vi "Demo Main_before_6_8_23_changes.vi"() -> ()   [LabVIEW 2022 SP3]
uses:
  Logo.ctl
  C:/Users/Public/OneDrive/Desktop/PMT program/SampleCodeLabView/Kinesis_with_LabVIEW_Examples_LV12 - v3/Thorlabs.MotionControl.Controls.dll
  Kinesis_with_LabVIEW_Examples_LV12 - v3/Thorlabs.MotionControl.Controls.dll
  <vilib>/Utility/file.llb/Write Delimited Spreadsheet (string).vi
  <vilib>/Utility/file.llb/Write Delimited Spreadsheet (I64).vi
  <vilib>/Utility/file.llb/Write Delimited Spreadsheet (DBL).vi
  C:/Users/Public/OneDrive/Desktop/PMT program/SampleCodeLabView/Kinesis_with_LabVIEW_Examples_LV12 - v3/ThorLabs.MotionControl.KCube.DCServoCLI.dll
  Kinesis_with_LabVIEW_Examples_LV12 - v3/ThorLabs.MotionControl.KCube.DCServoCLI.dll
  <vilib>/Analysis/NI_AALBase.lvlib
panel:
  in  "Save All Gate Data":bool
  out "ESD":i32=10000 caption="Steps\nAdded/Removed"
  in  "ES":i32 caption="Add /Remove \nSteps"
  out "Sweep Graph":u32[](graph)
  out "SM":i32 caption="Sweep\nMean"
  out "SN":i32 caption="Current Sweep Iteration"
  out "SND":i32 caption="Total No. of Sweeps"
  in  "Auto-Sweep":bool
  in  "P8":bool
  out "PC":i32 caption="Current \nPosition"
  out "WTD":i32=10000 caption="Wait Time (ms)\nRead Data"
  out "EPD":i32 caption="End Position\nRead Data"
  out "SPD":i32 caption="Start Position\nRead Data"
  out "SSD":i32 caption="Step Size\nRead Data"
  in  "SP":i32 caption="Start Position (degrees)\n Set Data"
  in  "WT":i32=10000 caption="Wait Time (ms)\n Set Data"
  in  "EP":i32 caption="End Position (degrees)\n Set Data"
  in  "P7":bool
  in  "SS":i32 caption="Step Size (degrees)\nSet Data"
  in  "Motor Controller\nSerialNumber":string="27261255"
  in  "KCubeDCServoControl":refnum<k24>(container)
  in  "Export":bool
  out "DB":u32[](array[numeric])
  out "OVL":bool caption="LED ON : Over Rang Data"
  out "OLD":i32
  out "GN":i32 caption="Gate Number"
  in  "Correction":bool=TRUE
  in  "Logo":T1
  out "Graph":u32[](graph)
  in  "Stop":bool
  in  "Start":bool
  in  "P6":bool
  out "RND":i32 caption="Read Number\nRead Data"
  in  "P5":bool
  in  "RN":i32=100 caption="Read Number\nSet Data"
  out "PowerD":i32 caption="Power\nRead Data"
  out "ITD":i32 caption="Internal Time\nRead Data"
  in  "P4":bool
  in  "P3":bool
  in  "IT":i32=100 caption="Internal Time\nSet Data"
  in  "P2":bool
  out "Handle Number":i32
  in  "P1":bool caption="Switch\nPower OFF/Power ON"
  in  "EXIT":bool
  # "pmt serial: 30430219"
  # "note: If you change angle between linear polarized light and half-wave plate by theta, the \npolarization after the wave plate is changed by twice theta. The code doesn't account for this.\nThis means we really need to go only to 180degrees, because at that point we have rotated the polarization by 360deg."
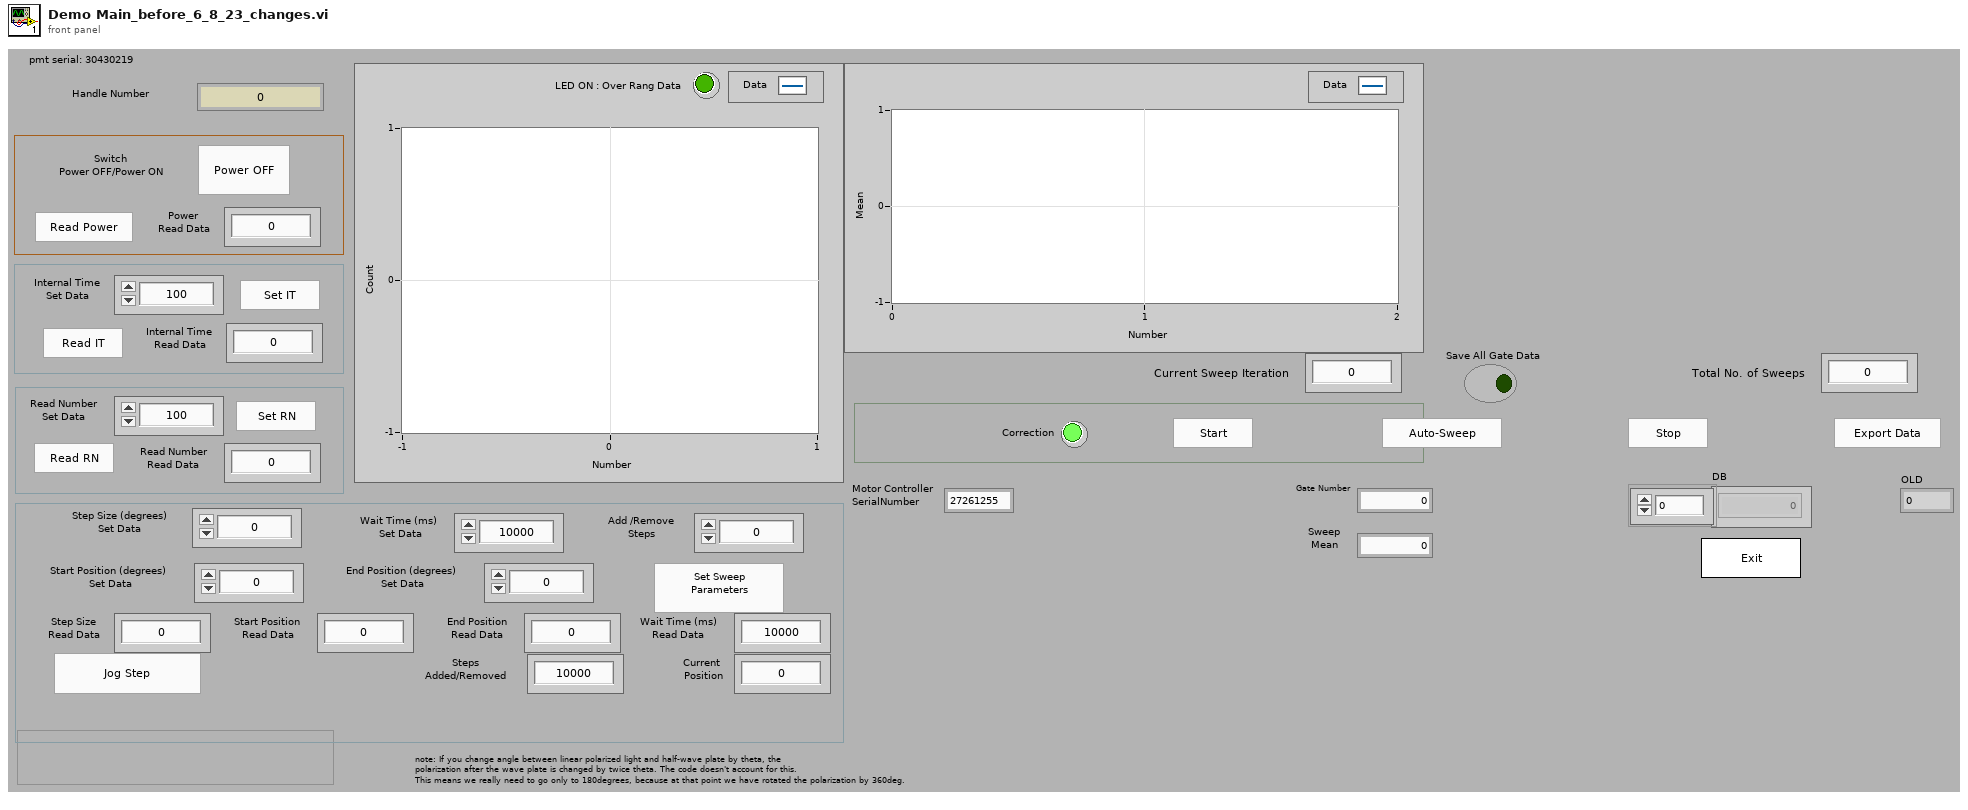
[diagram p1: front panel]
types:
  T1 = typedef "Logo.ctl" = bool
  T2 = enum8{"Enabled", "Disabled", "Disabled and Grayed Out"}
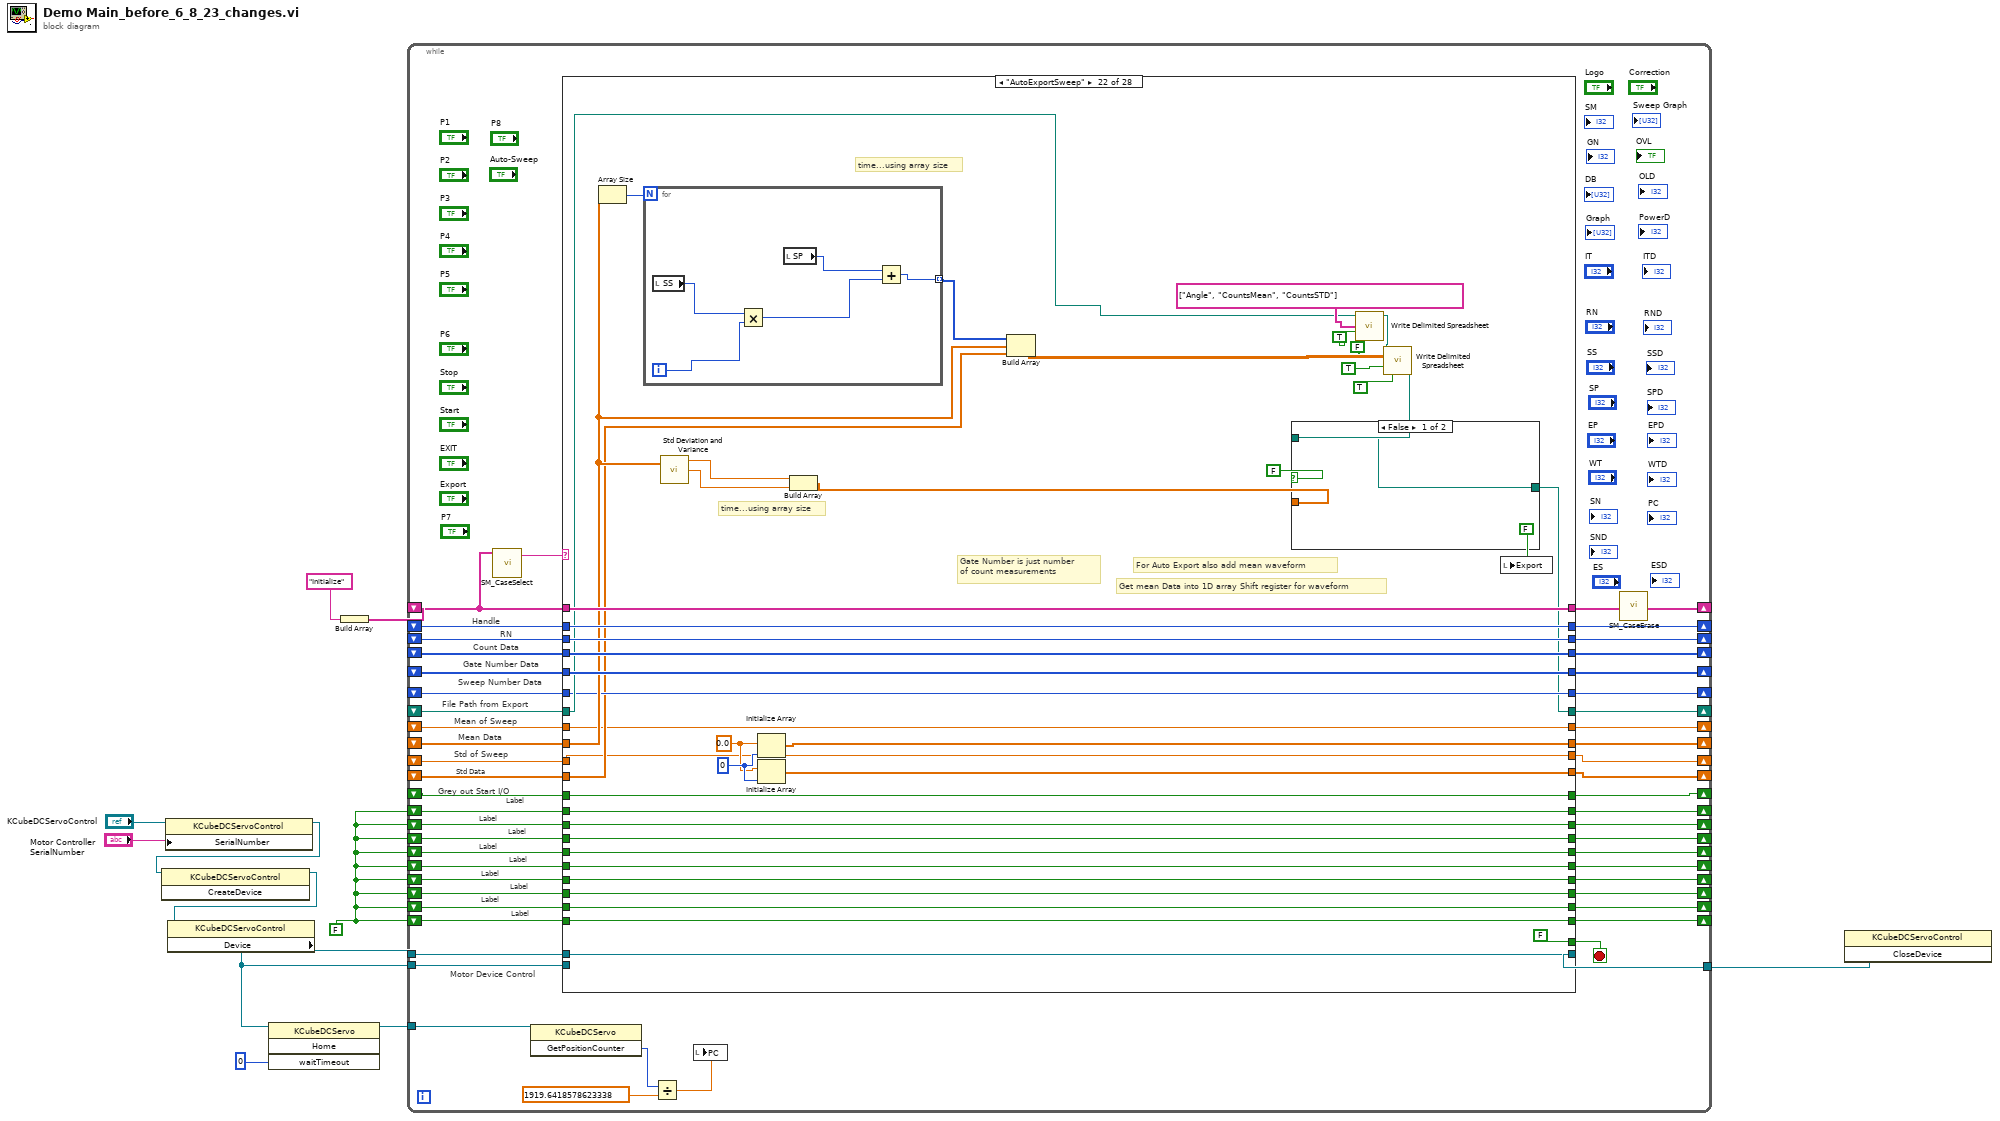
[diagram p0: block diagram]
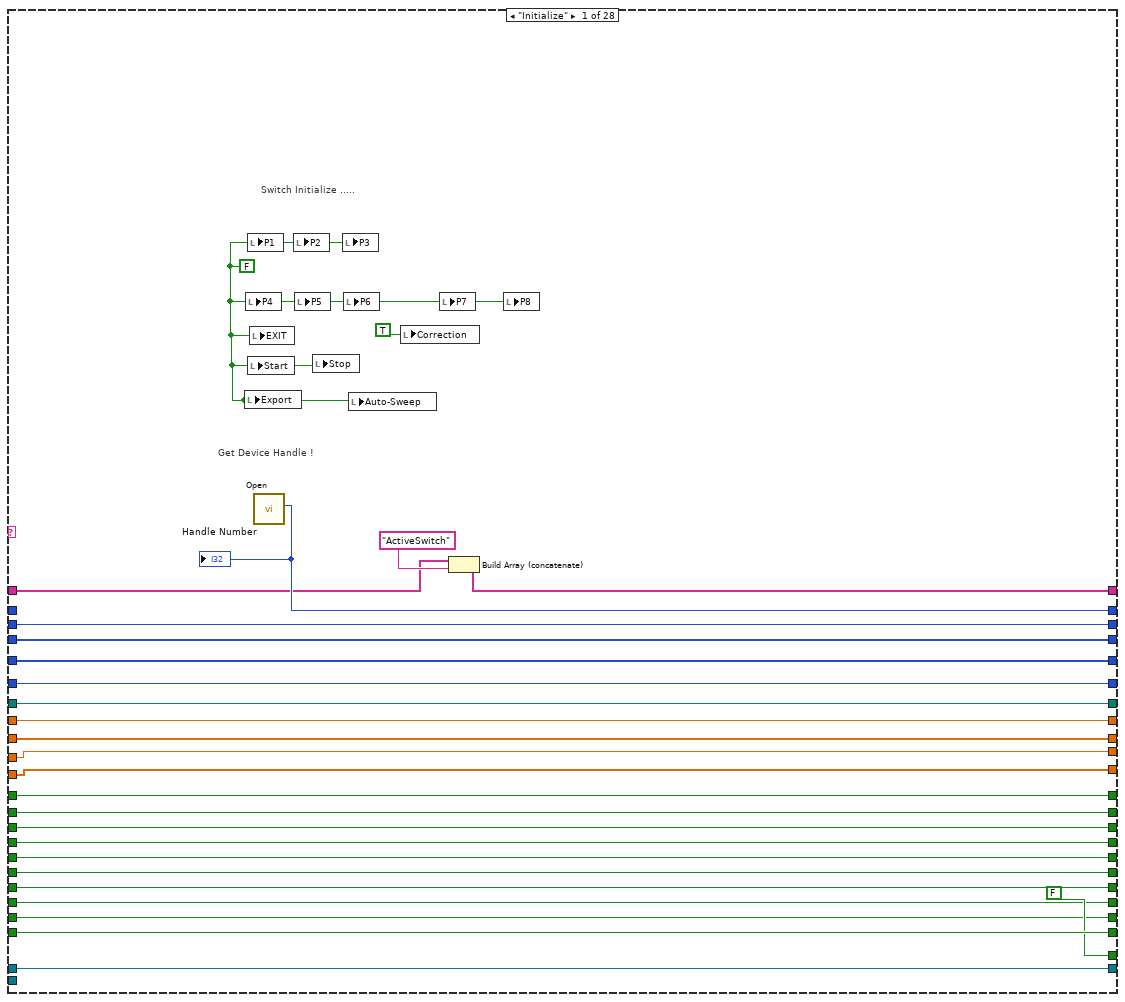
[diagram p2: hidden frame]
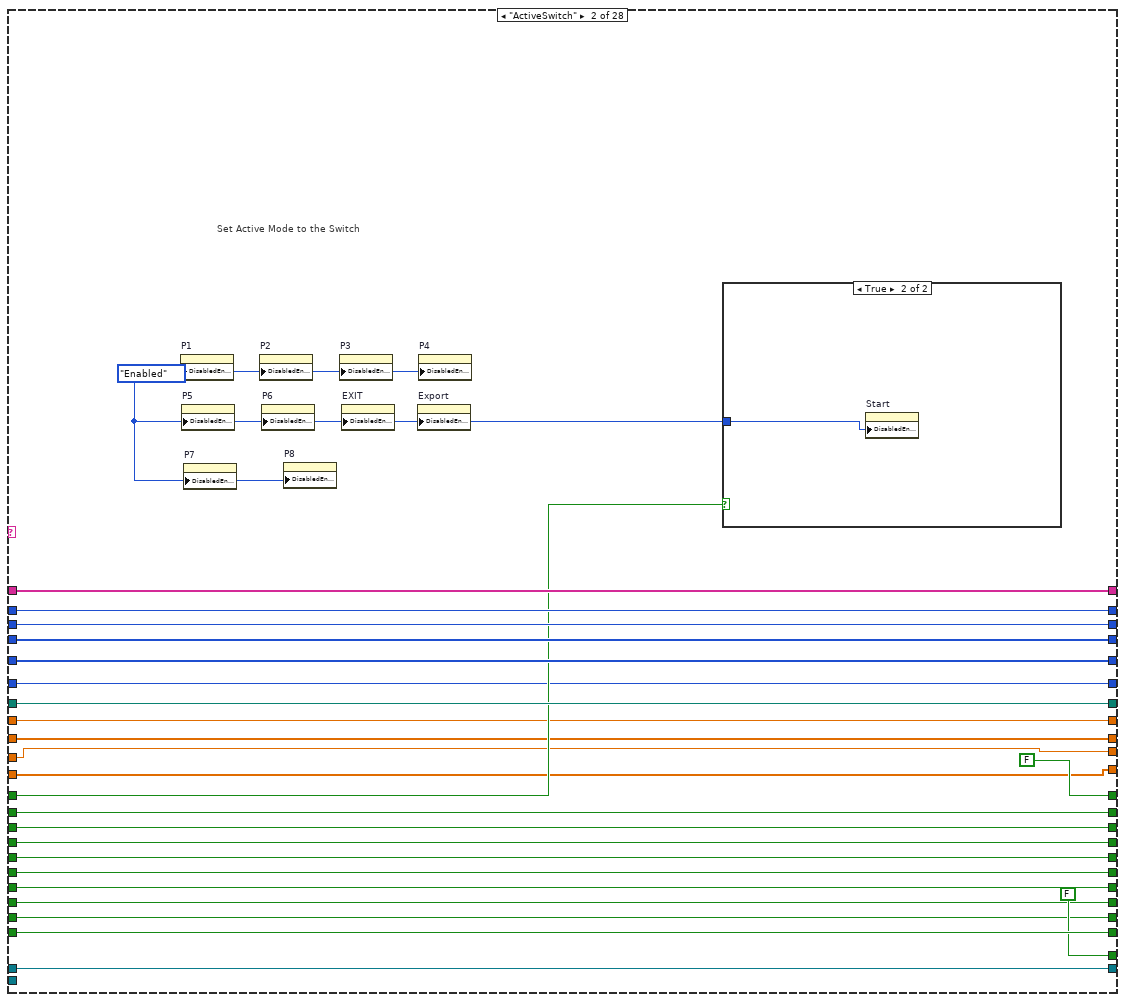
[diagram p3: hidden frame]
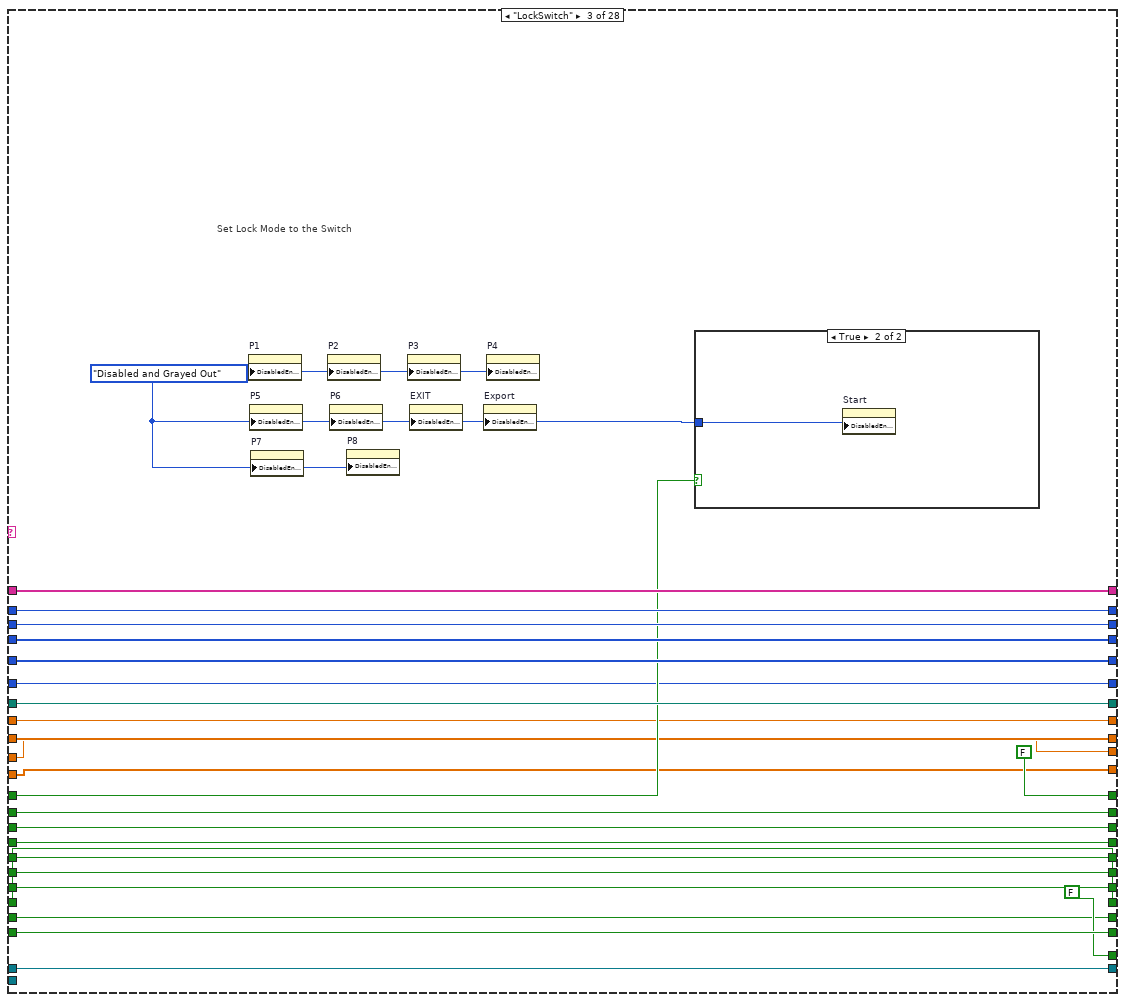
[diagram p5: hidden frame]
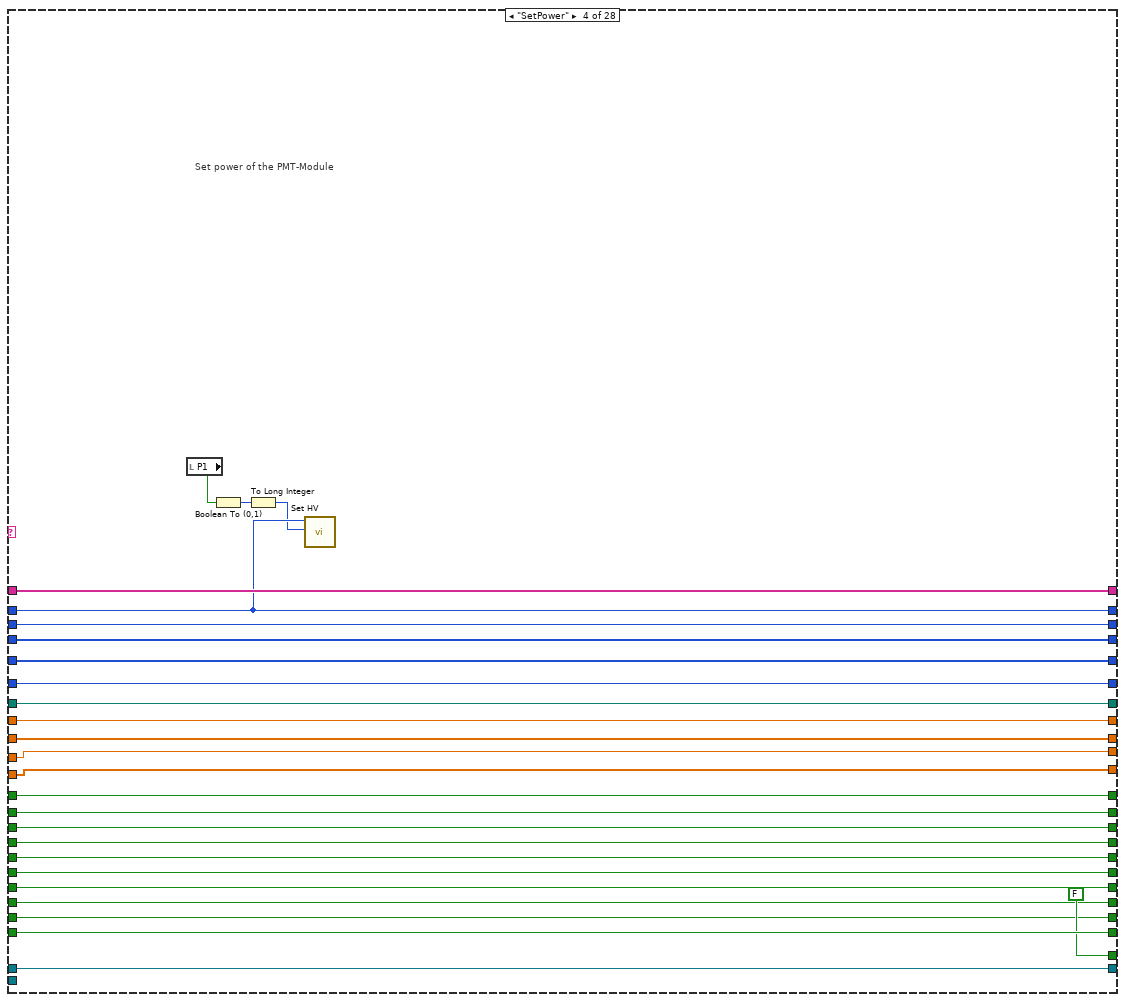
[diagram p7: hidden frame]
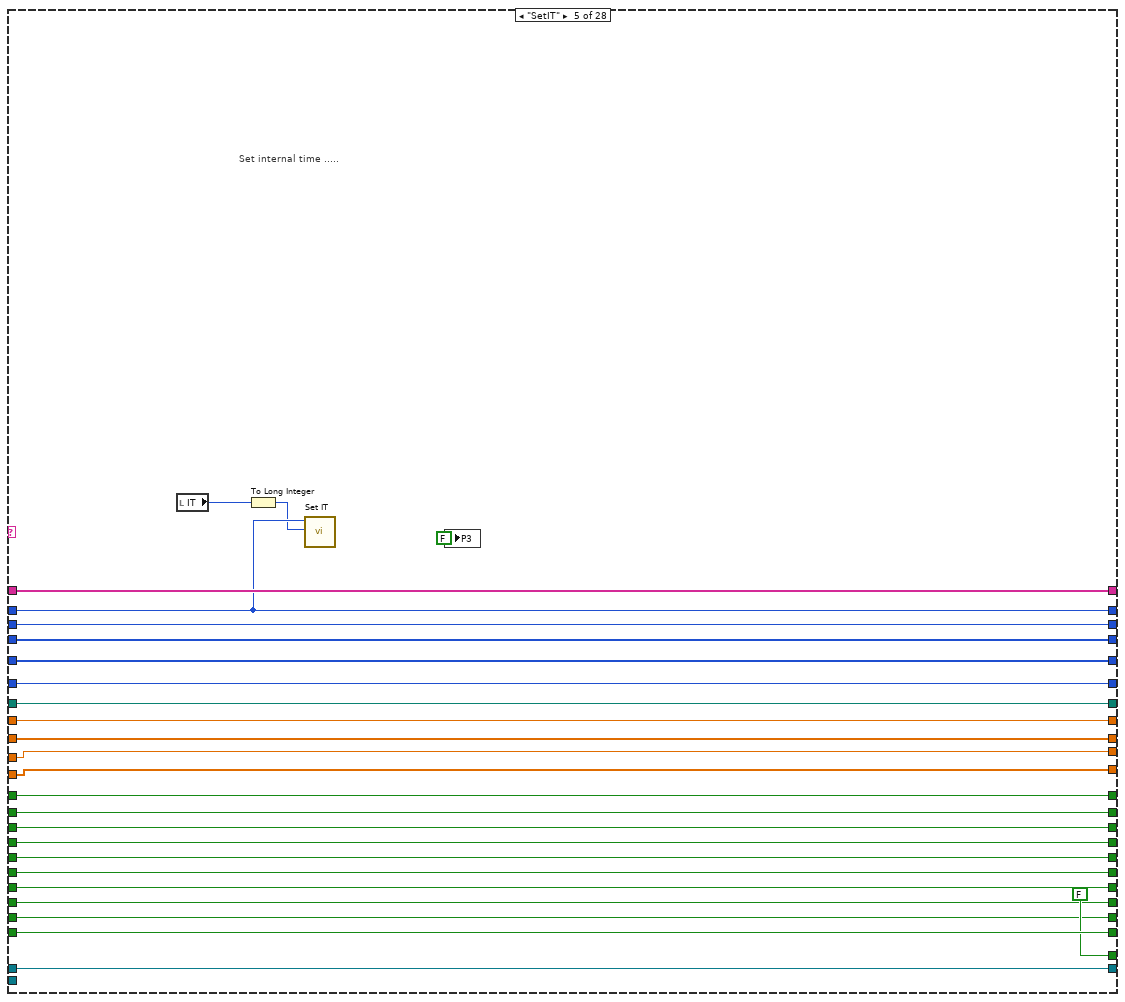
[diagram p8: hidden frame]
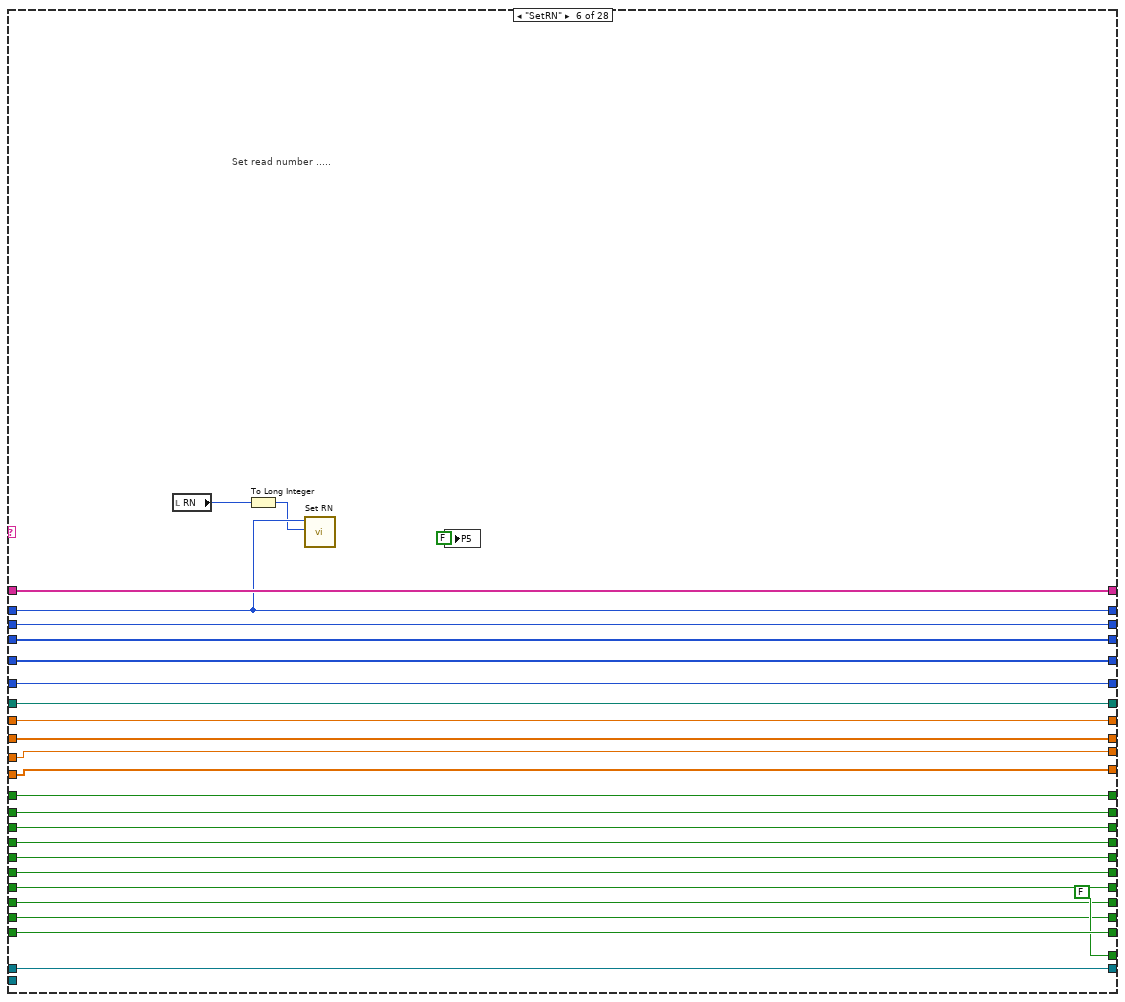
[diagram p9: hidden frame]
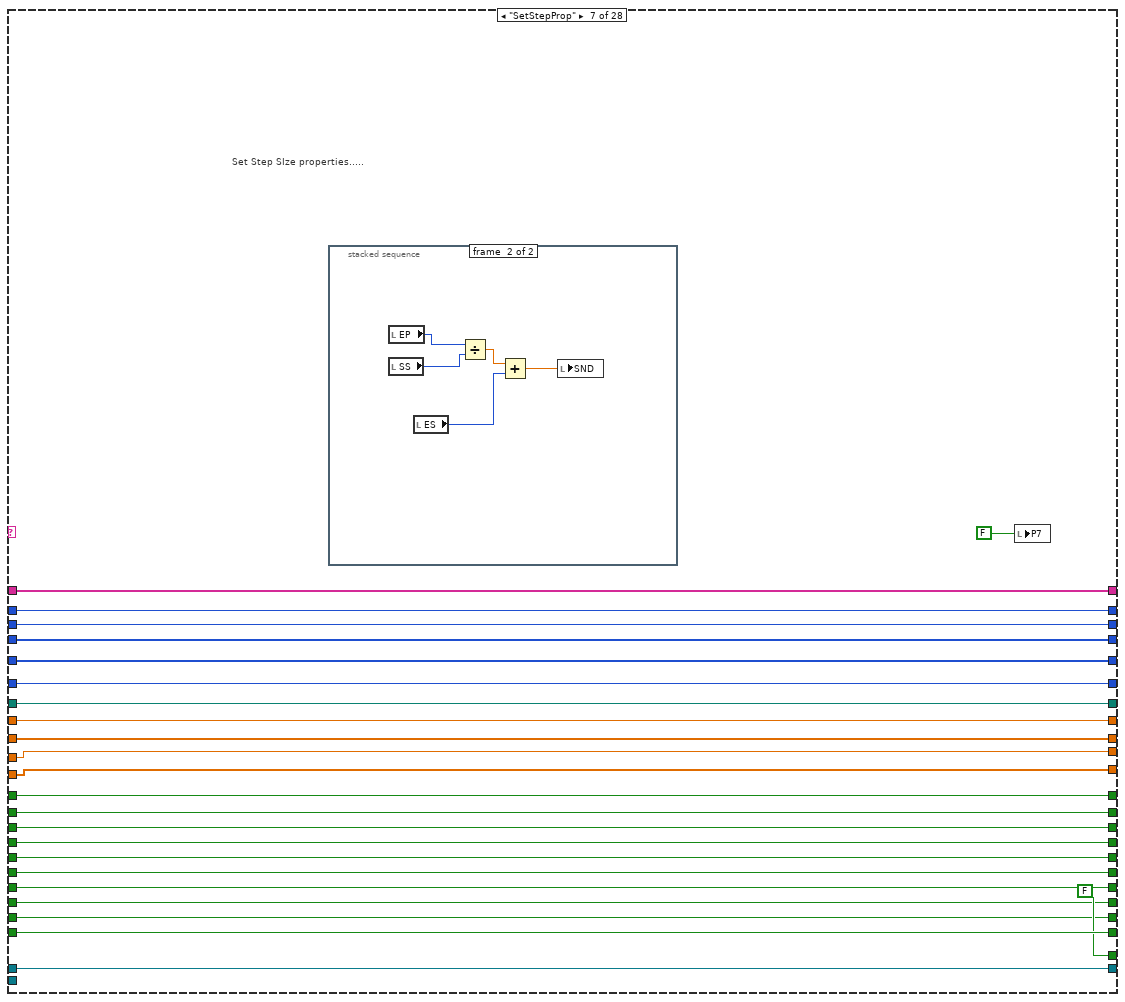
[diagram p10: hidden frame]
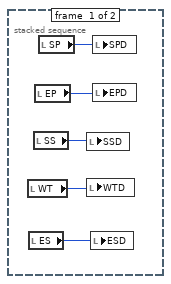
[diagram p11: hidden frame]
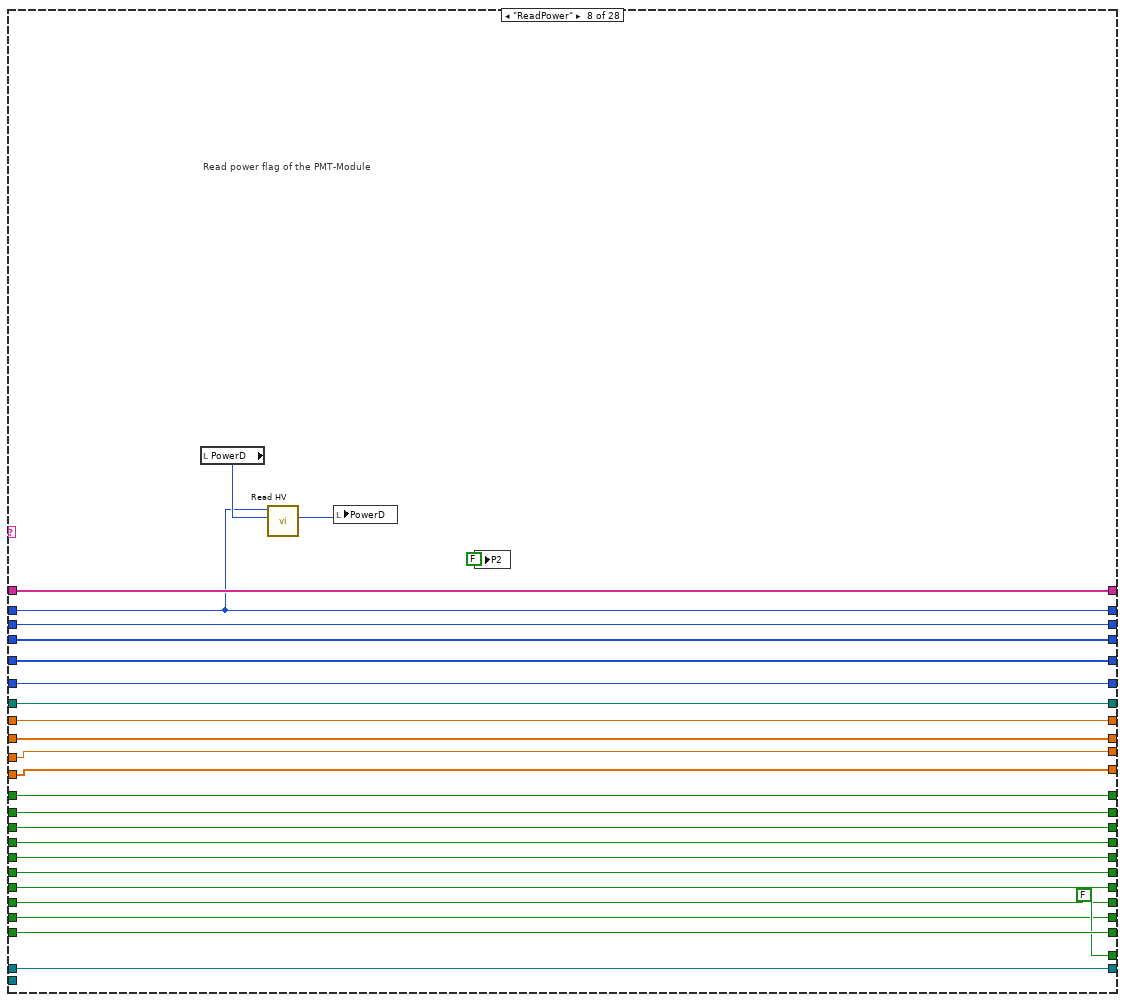
[diagram p12: hidden frame]
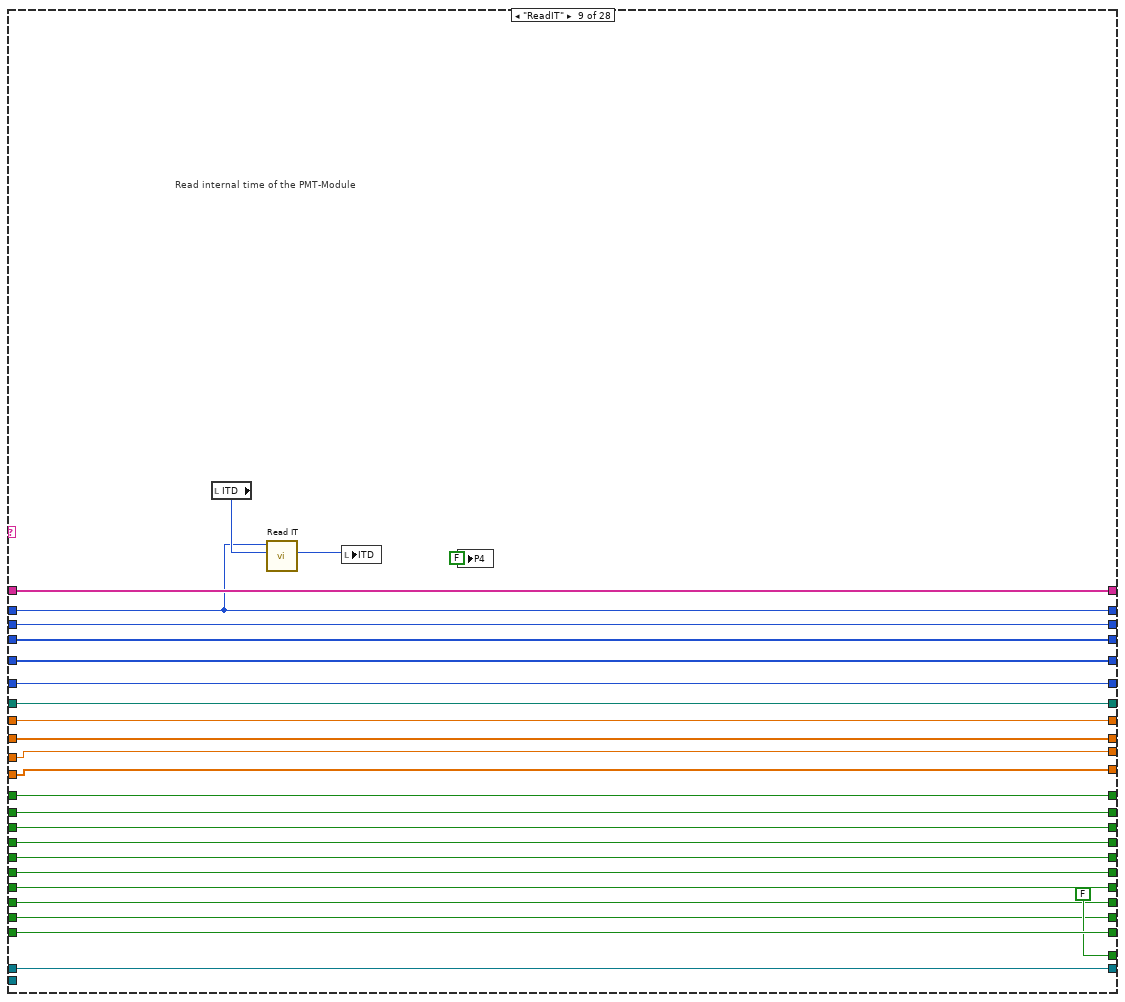
[diagram p13: hidden frame]
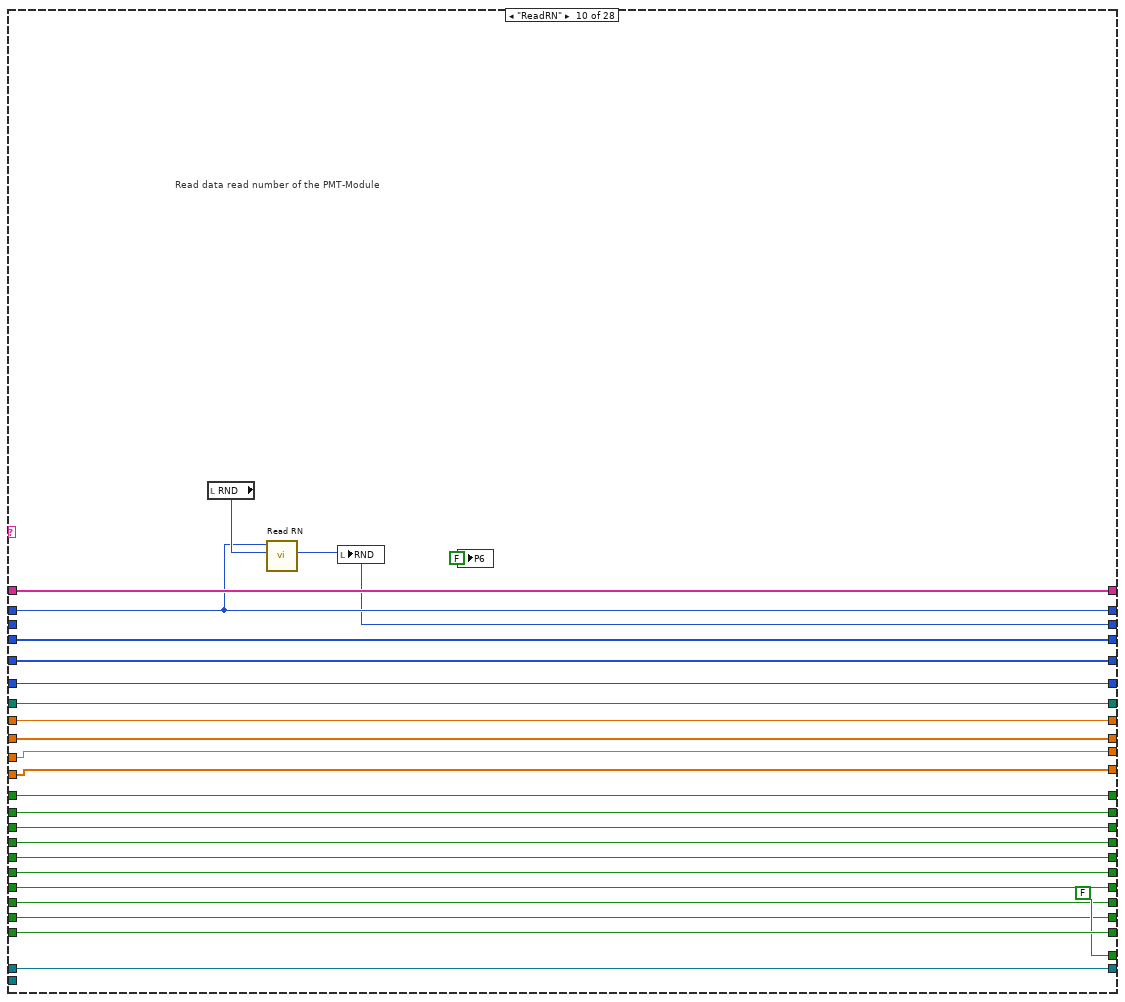
[diagram p14: hidden frame]
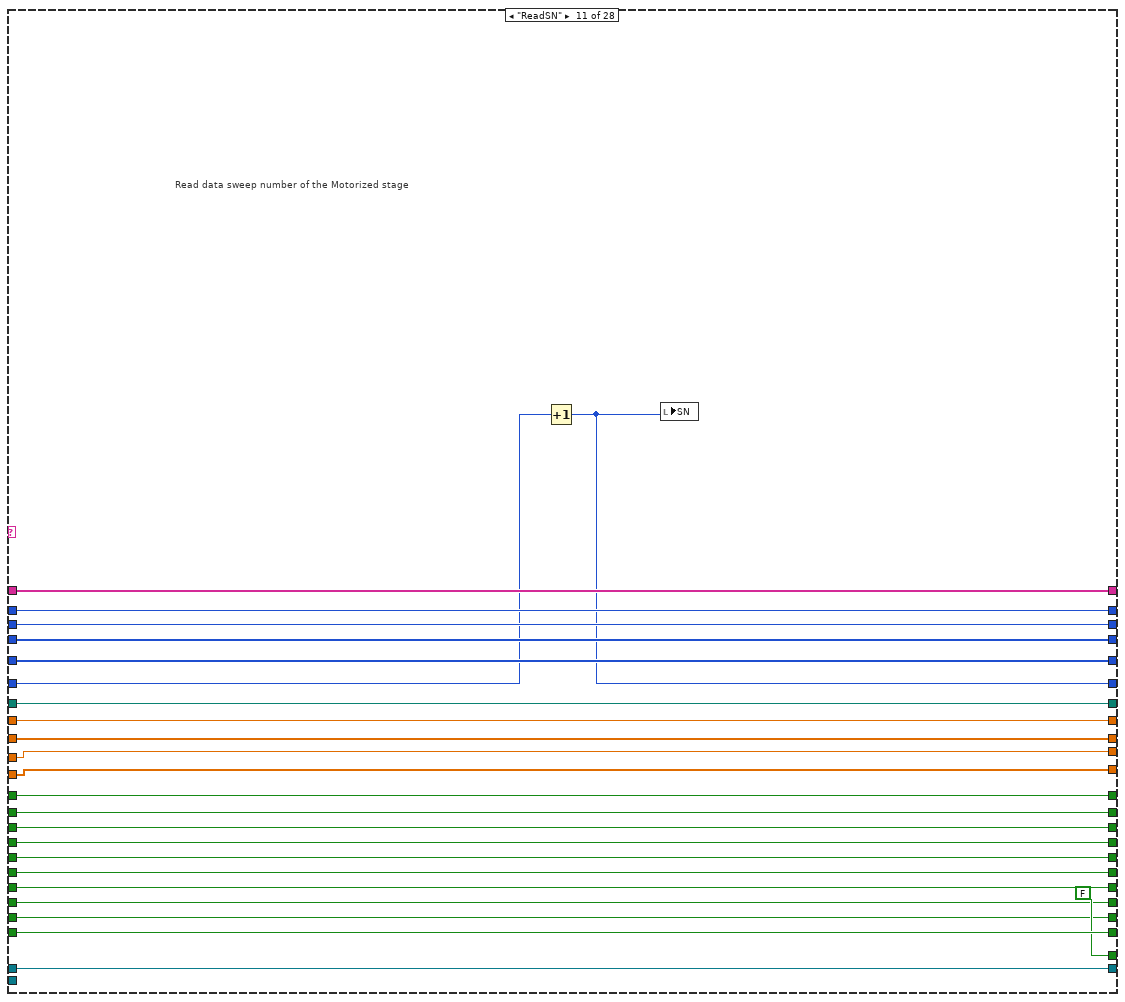
[diagram p15: hidden frame]
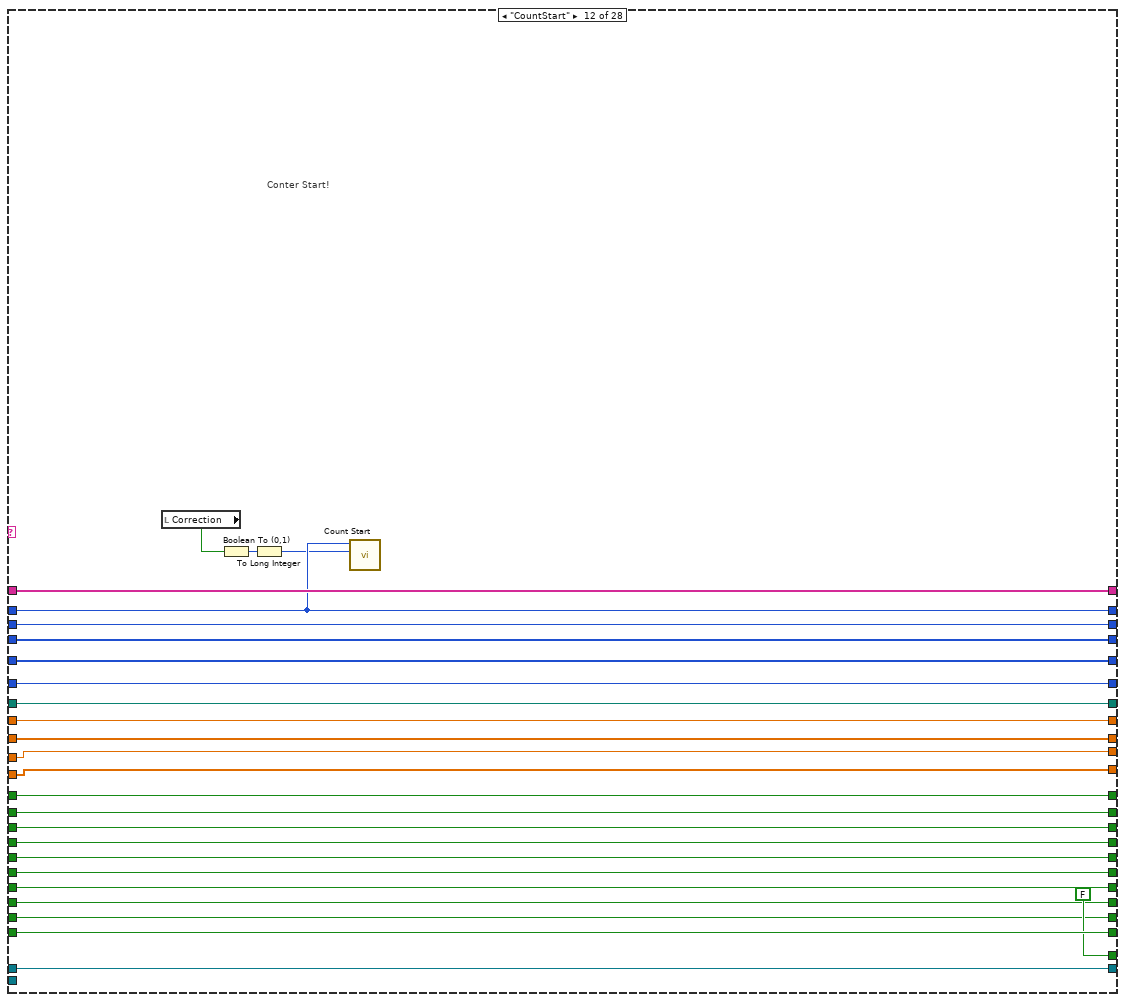
[diagram p16: hidden frame]
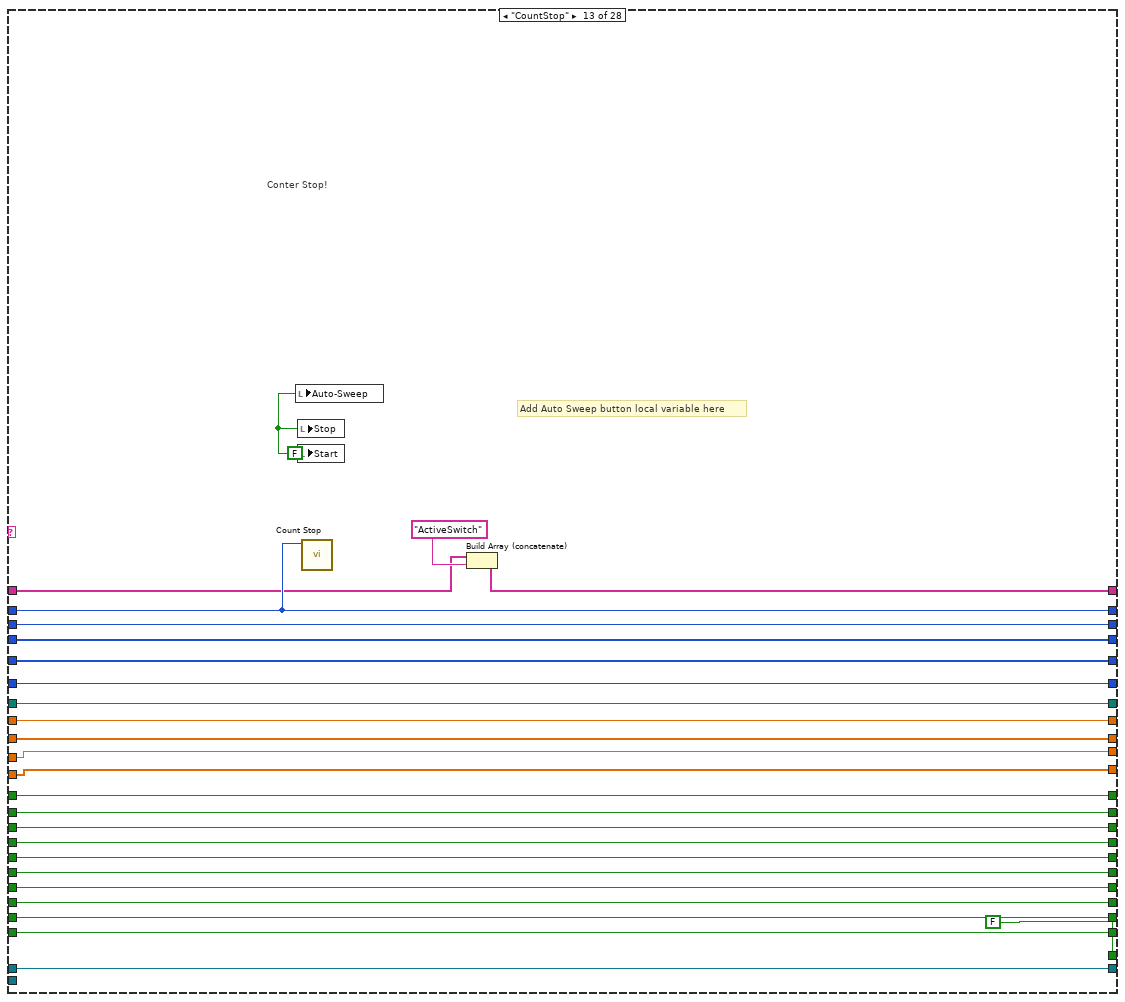
[diagram p17: hidden frame]
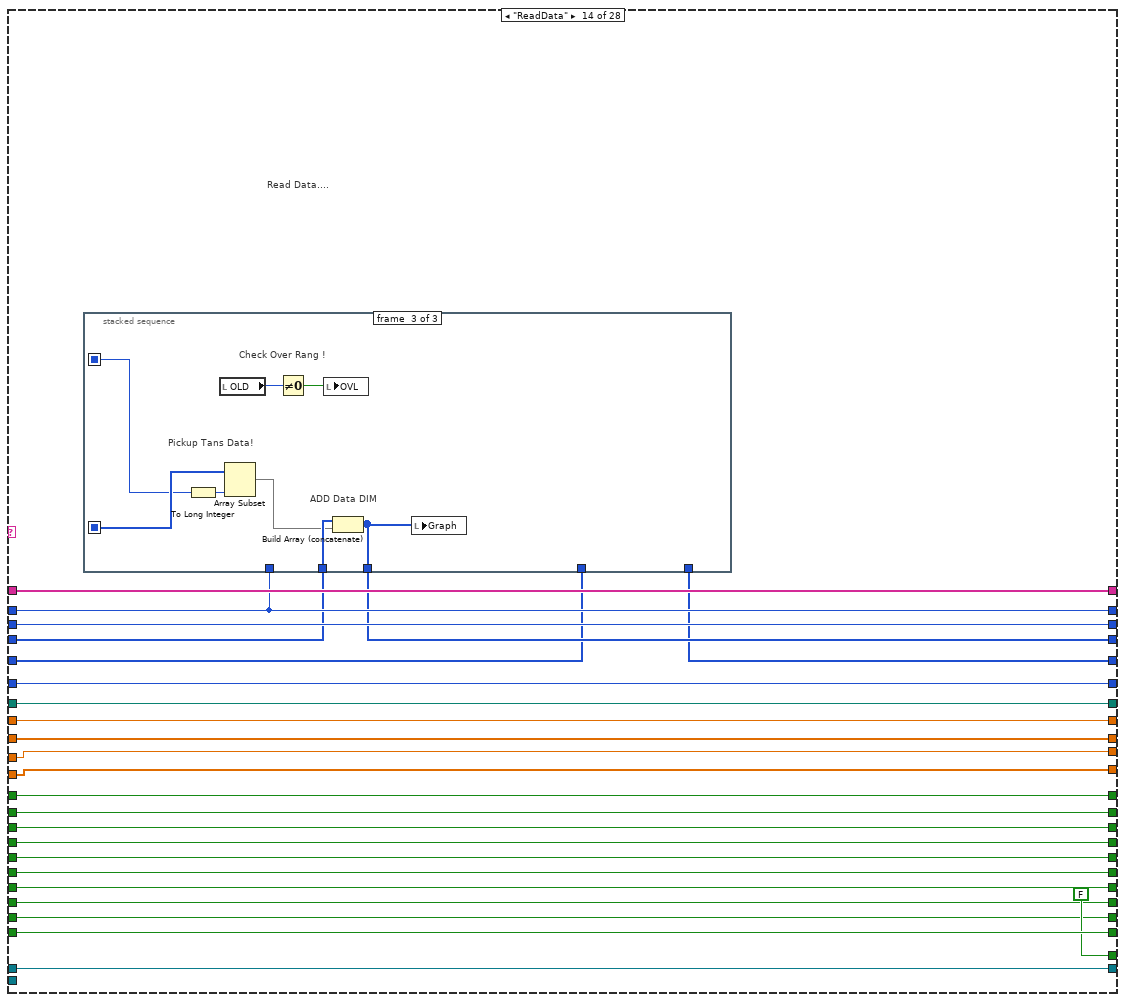
[diagram p18: hidden frame]
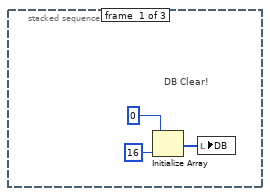
[diagram p19: hidden frame]
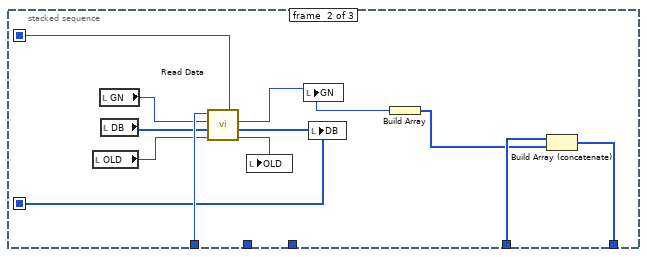
[diagram p20: hidden frame]
diagram:
  w10 = FALSE
  n1 = property class="KCubeDCServoControl"(reference="KCubeDCServoControl", "SerialNumber"="Motor Controller\nSerialNumber") -> (reference out=w8:refnum<k24>)  [unwired: 1 in, 1 out]
  n2 = invoke class="KCubeDCServoControl" method="CreateDevice"(reference=w8) -> (reference out=w1:refnum<k24>)  [unwired: 2 in, 2 out]
  n3 = property class="KCubeDCServoControl"(reference=w1) -> (reference out=w5:refnum<k24>, "Device"=w3:refnum<k24>)  [unwired: 1 in, 1 out]
  n4 = invoke class="KCubeDCServo" method="Home"(reference=w3, "waitTimeout"=0) -> (reference out=w2:refnum<k24>)  [unwired: 2 in, 3 out]
  n5 = Build Array("Initialize") -> (w11:string[])
  n6 = while {
    shift-right: [w47] -> _
    shift-left: w10 -> [w48]
    shift-right: [w49] -> _
    shift-left: w10 -> [w50]
    shift-right: [w51] -> _
    shift-left: w10 -> [w52]
    shift-right: [w53] -> _
    shift-left: w10 -> [w54]
    shift-right: [w55] -> _
    shift-left: _ -> [w56]
    shift-right: [w57] -> _
    shift-left: _ -> [w58]
    shift-right: [w59] -> _
    shift-left: _ -> [w60]
    shift-right: [w45] -> _
    shift-left: w10 -> [w46]
    shift-right: [w63] -> _
    shift-left: w10 -> [w64]
    shift-right: [w42] -> _
    shift-left: w11 -> [w61]
    shift-right: [w40] -> _
    shift-left: w10 -> [w41]
    shift-right: [w38] -> _
    shift-left: w10 -> [w39]
    shift-right: [w37] -> _
    shift-left: w10 -> [w36]
    tunnel: w5 -> [w33]
    tunnel: [w32] -> w6
    shift-right: [w35] -> _
    shift-left: _ -> [w34]
    tunnel: w3 -> [w31]
    shift-right: [w30] -> _
    shift-left: _ -> [w29]
    shift-right: [w28] -> _
    shift-left: _ -> [w27]
    tunnel: w2 -> [w26]
    shift-right: [w24] -> _
    shift-left: _ -> [w25]
    shift-right: [w23] -> _
    shift-left: _ -> [w22]
    shift-right: [w21] -> _
    shift-left: _ -> [w20]
    shift-right: [w15] -> _
    shift-left: _ -> [w16]
    shift-right: [w13] -> _
    shift-left: _ -> [w14]
    stop <- w44 stop-if-true
    # "Std Data"
    # "Std of Sweep"
    # "Mean Data"
    # "Mean of Sweep"
    # "Sweep Number Data"
    # "Grey out Start I/O"
    # "Motor Device Control"
    # "File Path from Export"
    # "Gate Number Data"
    # "Label"
    # "Label"
    # "Label"
    # "Label"
    # "Label"
    # "Label"
    # "Label"
    # "Label"
    # "Label"
    # "Count Data"
    # "RN"
    # "Handle"
    n7 = call "SM_CaseSelect.vi"("Input"=w61) -> ("Case"=w62:string)  [unwired: 10 out]
    n8 = invoke class="KCubeDCServo" method="GetPositionCounter"(reference=w26) -> ("GetPositionCounter"=w18:i32)  [unwired: 2 in, 2 out]
    n9 = case shown="\"AutoExportSweep\"" w62 {
      selector: w62 -> [_ _ _ _ _ _ _ _ _ _ _ _ _ _ _ _ _ _ _ _ _ _ _ _ _ _ w1015 _]
      tunnel: w64 -> [w91 w116 w142 w169 w195 w221 w245 w281 w307 w332 w356 w382 w408 w433 w480 w516 w544 w586 w626 w697 w736 w811 w853 w877 w911 w960 w1033 w1056]
      tunnel: [w91 w116 w142 w169 w195 w221 w245 w281 w307 w332 w356 w382 w408 w433 w480 w516 w544 w586 w626 w697 w736 w811 w853 w877 w911 w960 w1033 w1056] -> w63
      tunnel: w61 -> [w77 w115 w141 w168 w194 w220 w244 w280 w306 w331 w355 w381 w394 w432 w479 w504 w522 w573 w614 w708 w747 w822 w845 w890 w924 w948 w1032 w1055]
      tunnel: [w76 w115 w141 w168 w194 w220 w244 w280 w306 w331 w355 w381 w393 w432 w479 w503 w521 w574 w615 w708 w747 w822 w844 w890 w924 w945 w1032 w1055] -> w43
      tunnel: w60 -> [_ w103 w129 w156 w182 w208 w232 w267 w293 w319 w344 w369 w396 w421 w468 w505 w533 w576 w616 w707 w746 w821 w865 w889 w923 w959 w1031 w1043]
      tunnel: [w79 w103 w129 w156 w182 w208 w232 w267 w293 w319 w344 w369 w396 w421 w468 w505 w533 w576 w616 w707 w746 w821 w865 w889 w923 w959 w1031 w1043] -> w59
      tunnel: w58 -> [w90 w114 w140 w167 w193 w219 w243 w279 w305 _ w337 w380 w407 w431 w478 w515 w543 w571 w612 w706 w745 w820 w864 w888 w922 w958 w1030 w1054]
      tunnel: [w90 w114 w140 w167 w193 w219 w243 w279 w305 w317 w337 w380 w407 w431 w478 w515 w543 w571 w612 w706 w745 w820 w864 w888 w922 w958 w1030 w1054] -> w57
      tunnel: w56 -> [w89 w113 w139 w166 w192 w218 w242 w278 w304 w330 w354 w379 w406 w420 w463 _ _ w567 w610 w682 w731 w801 w863 w887 w921 w944 w1029 w1053]
      tunnel: [w89 w113 w139 w166 w192 w218 w242 w278 w304 w330 w354 w379 w406 w419 w463 w495 w531 w567 w610 w682 w731 w801 w863 w887 w921 w944 w1029 w1053] -> w55
      tunnel: w54 -> [w88 w112 w138 w165 w191 w217 w241 w277 w303 w329 w353 w378 w405 w430 w477 w514 w542 w585 w625 w705 w744 w819 w861 w885 w919 w957 w1028 w1052]
      tunnel: [w88 w112 w138 w165 w191 w217 w241 w277 w303 w329 w353 w378 w405 w430 w477 w514 w542 w585 w625 w705 w744 w819 w861 w885 w919 w957 w1028 w1052] -> w53
      tunnel: w52 -> [w87 w111 w137 w164 w190 w216 w240 w276 w302 w328 w352 w377 w404 w429 w476 w513 w541 w584 w624 w704 w743 w818 w860 w884 w918 w956 w1027 w1051]
      tunnel: [w87 w111 w137 w164 w190 w216 w240 w276 w302 w328 w352 w377 w404 w429 w476 w513 w541 w584 w624 w704 w743 w818 w860 w884 w918 w956 w1027 w1051] -> w51
      tunnel: w50 -> [w86 w110 w136 w163 w189 w215 w239 w275 w301 w327 w351 w376 w403 w428 w475 w512 w540 w583 w623 w703 w742 w817 w859 w883 w917 w955 w1026 w1050]
      tunnel: [w86 w110 w136 w163 w189 w215 w239 w275 w301 w327 w351 w376 w403 w428 w475 w512 w540 w583 w623 w703 w742 w817 w859 w883 w917 w955 w1026 w1050] -> w49
      tunnel: w48 -> [w85 w109 w135 w162 w188 w214 w238 w274 w300 w326 w350 w375 w402 w427 w474 w511 w539 w582 w622 w702 w741 w816 w858 w882 w916 w954 w1025 w1049]
      tunnel: [w85 w109 w135 w162 w188 w214 w238 w274 w300 w326 w350 w375 w402 w427 w474 w511 w539 w582 w622 w702 w741 w816 w858 w882 w916 w954 w1025 w1049] -> w47
      tunnel: w46 -> [w84 w108 w134 w161 w187 w213 w237 w273 w299 w325 w349 w374 w401 w426 w473 w510 w538 w581 w621 w701 w740 w815 w857 w881 w915 w953 w1024 w1048]
      tunnel: [w84 w108 w134 w161 w187 w213 w237 w273 w299 w325 w349 w374 w401 w426 w473 w510 w538 w581 w621 w701 w740 w815 w857 w881 w915 w953 w1024 w1048] -> w45
      tunnel: [FALSE FALSE FALSE FALSE FALSE FALSE FALSE FALSE FALSE FALSE FALSE FALSE FALSE FALSE FALSE FALSE FALSE FALSE FALSE FALSE FALSE FALSE FALSE FALSE FALSE FALSE FALSE TRUE] -> w44
      tunnel: w41 -> [w80 w104 w130 w157 w183 w209 w233 w269 w295 w321 w345 w370 w397 w422 w469 w506 w534 w577 w617 w700 w739 w814 w856 w880 w914 w949 w1020 w1044]
      tunnel: [w80 w104 w130 w157 w183 w209 w233 w269 w295 w321 w345 w370 w397 w422 w469 w506 w534 w577 w617 w700 w739 w814 w856 w880 w914 w949 w1020 w1044] -> w40
      tunnel: w39 -> [w82 w106 w132 w159 w185 w211 w235 w271 w297 w323 w347 w372 w399 w424 w471 w508 w536 w579 w619 w699 w738 w813 w855 w879 w913 w951 w1022 w1046]
      tunnel: [w82 w106 w132 w159 w185 w211 w235 w271 w297 w323 w347 w372 w399 w424 w471 w508 w536 w579 w619 w699 w738 w813 w855 w879 w913 w951 w1022 w1046] -> w38
      tunnel: [w81 w105 w131 w158 w184 w210 w234 w270 w296 w322 w346 w371 w398 w423 w470 w507 w535 w578 w618 w698 w737 w812 w854 w878 w912 w950 w1021 w1045] -> w37
      tunnel: w36 -> [w81 w105 w131 w158 w184 w210 w234 w270 w296 w322 w346 w371 w398 w423 w470 w507 w535 w578 w618 w698 w737 w812 w854 w878 w912 w950 w1021 w1045]
      tunnel: [w75 w102 w128 w152 w178 w204 w231 w264 w290 w316 w343 w365 w392 w418 w462 w495 w531 w566 w609 w677 w717 w796 w862 w886 w920 w943 w1014 w1042] -> w35
      tunnel: w34 -> [w75 w102 w128 w152 w178 w204 w231 w264 w290 w316 w343 w365 w392 w417 w462 _ _ w566 w609 w677 w717 w796 w862 w886 w920 w943 w1014 w1042]
      tunnel: w33 -> [w74 w101 w127 w151 w177 w203 w230 w263 w289 w315 w342 w364 w391 w416 w467 w494 w530 w565 w608 w679 w729 w798 w852 w876 w910 w942 w1013 w1041]
      tunnel: [w74 w101 w127 w151 w177 w203 w230 w263 w289 w315 w342 w364 w391 w416 w467 w494 w530 w565 w608 w679 w729 w798 w852 w876 w910 w942 w1013 w1041] -> w32
      tunnel: w31 -> [_ _ _ _ _ _ _ _ _ _ _ _ _ _ _ _ _ _ _ _ _ _ _ w873 w907 _ _ _]
      tunnel: [w73 w100 w126 w150 w176 w202 w228 w262 w288 w314 w341 w363 w390 w415 w466 w493 w529 w564 w607 w670 w727 w780 w841 w874 w908 w941 w1012 w1040] -> w30
      tunnel: w29 -> [w73 w100 w126 w150 w176 w202 w228 w262 w288 w314 w341 w363 w390 w415 w466 w493 w529 w564 w607 w670 w723 w794 _ w874 w908 w941 w1012 w1040]
      tunnel: [w72 FALSE FALSE w149 w175 w201 w227 w261 w287 w313 w340 w362 w389 w414 w465 w492 TRUE w563 w606 w672 w726 w795 w850 w872 w906 w940 w1011 w1039] -> w28
      tunnel: w27 -> [w72 w99 w125 w149 w175 w201 w227 w261 w287 w313 w340 w362 w389 w414 w465 w492 _ w563 _ w672 w726 w795 w850 w872 w906 w940 w1011 w1039]
      tunnel: w25 -> [w70 w96 w122 w148 w174 w200 w226 w260 w286 w312 w335 w361 w388 w413 w464 w491 w527 w562 w605 w671 w722 w791 _ w868 w905 w939 w1010 w1038]
      tunnel: [w70 w96 w122 w148 w174 w200 w226 w260 w286 w312 w336 w361 w388 w413 w464 w491 w527 w562 w605 w671 w722 w791 w842 w868 w905 w939 w1010 w1038] -> w24
      tunnel: [w69 w95 w121 w147 w173 w199 w225 w259 w285 w311 w339 w360 w387 w412 w461 w490 w526 w561 w602 w669 w725 w784 w849 w870 w904 w938 w1009 w1037] -> w23
      tunnel: w22 -> [w69 w95 w121 w147 w173 w199 w225 w259 w285 w311 w339 w360 w387 w412 w461 w490 w526 w561 w602 w669 _ w784 w849 w870 w904 w938 w1009 w1037]
      tunnel: [w68 w94 w120 w146 w172 w198 w224 w258 w284 w310 w338 w359 w386 w411 w460 w489 w525 w560 w601 w668 w724 w790 w843 w869 w903 w937 w1008 w1036] -> w21
      tunnel: w20 -> [w68 w94 w120 w146 w172 w198 w224 w258 w284 w310 w338 w359 w386 w411 w459 w489 w525 w560 w601 w668 w724 w792 w843 w869 w903 w937 w1008 w1036]
      tunnel: w16 -> [w67 w93 w119 w145 w171 w197 w223 w257 w283 w309 w334 w358 w384 w410 w458 w488 w518 w559 w599 w667 w716 w786 w839 w867 w902 w936 w1007 w1035]
      tunnel: [w67 w93 w119 w145 w171 w197 w223 w257 w283 w309 w334 w358 w384 w410 w456 w488 w518 w559 w599 w667 w716 w787 w839 w867 w902 w936 w1007 w1035] -> w15
      tunnel: w14 -> [w66 w92 w118 w144 w170 w196 w222 w256 w282 w308 w333 w357 w383 w409 w457 w487 w517 w558 w598 w666 _ w783 w838 w866 w901 w935 w1006 w1034]
      tunnel: [w66 w92 w118 w144 w170 w196 w222 w256 w282 w308 w333 w357 w383 w409 w457 w487 w517 w558 w598 w666 w715 w783 w838 w866 w901 w935 w1006 w1034] -> w13
      frame "Initialize" {
        w71 = FALSE ("P1")
        # "Get Device Handle !"
        # "Switch Initialize ....."
        n10 = local write "Export"(w71) -> ()
        n11 = local write "P4"(w71) -> ()
        n12 = local write "P1"(w71) -> ()
        n13 = local write "Start"(w71) -> ()
        n14 = local write "EXIT"(w71) -> ()
        n15 = call "Open.vi"() -> ("Handle Number"=w79:i32)  [unwired: 10 in, 1 out]
        "Handle Number" <- w79
        n16 = local write "P2"(w71) -> ()
        n17 = local write "P5"(w71) -> ()
        n18 = local write "Stop"(w71) -> ()
        n19 = local write "P3"(w71) -> ()
        n20 = local write "P6"(w71) -> ()
        n21 = local write "Auto-Sweep"(w71) -> ()
        n22 = local write "Correction"(TRUE ("P1")) -> ()
        n23 = local write "P7"(w71) -> ()
        n24 = Build Array (concatenate)(w77, "ActiveSwitch") -> (w76:string[])
        n25 = local write "P8"(w71) -> ()
      }
      frame "ActiveSwitch" {
        w97 = T2."Enabled" ("無効")
        # "Set Active Mode to the Switch"
        n26 = property on="P1" class="Bool (strict)"("DisabledEnum"=w97) -> ()  [unwired: 2 in, 2 out]
        n27 = property on="P5" class="Bool (strict)"("DisabledEnum"=w97) -> ()  [unwired: 2 in, 2 out]
        n28 = property on="P7" class="Bool (strict)"("DisabledEnum"=w97) -> ()  [unwired: 2 in, 2 out]
        n29 = property on="P2" class="Bool (strict)"("DisabledEnum"=w97) -> ()  [unwired: 2 in, 2 out]
        n30 = property on="P6" class="Bool (strict)"("DisabledEnum"=w97) -> ()  [unwired: 2 in, 2 out]
        n31 = property on="P8" class="Bool (strict)"("DisabledEnum"=w97) -> ()  [unwired: 2 in, 2 out]
        n32 = property on="P3" class="Bool (strict)"("DisabledEnum"=w97) -> ()  [unwired: 2 in, 2 out]
        n33 = property on="EXIT" class="Bool (strict)"("DisabledEnum"=w97) -> ()  [unwired: 2 in, 2 out]
        n34 = property on="Export" class="Bool (strict)"("DisabledEnum"=w97) -> ()  [unwired: 2 in, 2 out]
        n35 = property on="P4" class="Bool (strict)"("DisabledEnum"=w97) -> ()  [unwired: 2 in, 2 out]
        n36 = case shown="True" w99 {
          tunnel: w97 -> [_ w117]
          frame False {
          }
          frame True {
            n37 = property on="Start" class="Bool (strict)"("DisabledEnum"=w117) -> ()  [unwired: 2 in, 2 out]
          }
        }
      }
      frame "LockSwitch" {
        w123 = T2."Disabled and Grayed Out" ("無効")
        # "Set Lock Mode to the Switch"
        n38 = property on="P1" class="Bool (strict)"("DisabledEnum"=w123) -> ()  [unwired: 2 in, 2 out]
        n39 = property on="P5" class="Bool (strict)"("DisabledEnum"=w123) -> ()  [unwired: 2 in, 2 out]
        n40 = property on="P7" class="Bool (strict)"("DisabledEnum"=w123) -> ()  [unwired: 2 in, 2 out]
        n41 = property on="P2" class="Bool (strict)"("DisabledEnum"=w123) -> ()  [unwired: 2 in, 2 out]
        n42 = property on="P6" class="Bool (strict)"("DisabledEnum"=w123) -> ()  [unwired: 2 in, 2 out]
        n43 = property on="P8" class="Bool (strict)"("DisabledEnum"=w123) -> ()  [unwired: 2 in, 2 out]
        n44 = property on="P3" class="Bool (strict)"("DisabledEnum"=w123) -> ()  [unwired: 2 in, 2 out]
        n45 = property on="EXIT" class="Bool (strict)"("DisabledEnum"=w123) -> ()  [unwired: 2 in, 2 out]
        n46 = property on="Export" class="Bool (strict)"("DisabledEnum"=w123) -> ()  [unwired: 2 in, 2 out]
        n47 = property on="P4" class="Bool (strict)"("DisabledEnum"=w123) -> ()  [unwired: 2 in, 2 out]
        n48 = case shown="True" w125 {
          tunnel: w123 -> [_ w143]
          frame False {
          }
          frame True {
            n49 = property on="Start" class="Bool (strict)"("DisabledEnum"=w143) -> ()  [unwired: 2 in, 2 out]
          }
        }
      }
      frame "SetPower" {
        # "Set power of the PMT-Module"
        n50 = local read "P1"() -> (w155:bool)
        n51 = Boolean To (0,1)(Boolean=w155) -> (0, 1=w154:i16)
        n52 = To Long Integer(number=w154) -> (32bit integer=w153:i32)
        n53 = call "Set HV.vi"("HV"=w153, "handle"=w156) -> ()  [unwired: 8 in, 2 out]
      }
      frame "SetIT" {
        # "Set internal time ....."
        n54 = local read "IT"() -> (w180:i32)
        n55 = To Long Integer(number=w180) -> (32bit integer=w181:i32)
        n56 = call "Set IT.vi"("IT"=w181, "handle"=w182) -> ()  [unwired: 8 in, 2 out]
        n57 = local write "P3"(FALSE ("P3")) -> ()
      }
      frame "SetRN" {
        # "Set read number ....."
        n58 = local read "RN"() -> (w206:i32)
        n59 = To Long Integer(number=w206) -> (32bit integer=w207:i32)
        n60 = call "Set RN.vi"("RN"=w207, "handle"=w208) -> ()  [unwired: 8 in, 2 out]
        n61 = local write "P5"(FALSE ("P3")) -> ()
      }
      frame "SetStepProp" {
        # "Set Step SIze properties....."
        n62 = stacked-sequence {
          frame #0 {
            n63 = local read "WT"() -> (w247:i32)
            n64 = local read "ES"() -> (w246:i32)
            n65 = local read "SS"() -> (w248:i32)
            n66 = local read "EP"() -> (w249:i32)
            n67 = local read "SP"() -> (w250:i32)
            n68 = local write "SSD"(w248) -> ()
            n69 = local write "WTD"(w247) -> ()
            n70 = local write "ESD"(w246) -> ()
            n71 = local write "SPD"(w250) -> ()
            n72 = local write "EPD"(w249) -> ()
          }
          frame #1 {
            n73 = local read "EP"() -> (w255:i32)
            n74 = local read "SS"() -> (w254:i32)
            n75 = local read "ES"() -> (w252:i32)
            n76 = Divide(x=w255, y=w254) -> (x/y=w253:dbl)
            n77 = Add(x=w253, y=w252) -> (x+y=w251:dbl)
            n78 = local write "SND"(w251) -> ()
          }
        }
        n79 = local write "P7"(FALSE) -> ()
      }
      frame "ReadPower" {
        # "Read power flag of the PMT-Module"
        n80 = local read "PowerD"() -> (w268:i32)
        n81 = call "Read HV.vi"("HV"=w268, "handle"=w267) -> ("HV out"=w266:i32)  [unwired: 7 in, 2 out]
        n82 = local write "PowerD"(w266) -> ()
        n83 = local write "P2"(FALSE ("P2")) -> ()
      }
      frame "ReadIT" {
        # "Read internal time of the PMT-Module"
        n84 = local read "ITD"() -> (w294:i32)
        n85 = call "Read IT.vi"("IT"=w294, "handle"=w293) -> ("IT out"=w292:i32)  [unwired: 7 in, 2 out]
        n86 = local write "ITD"(w292) -> ()
        n87 = local write "P4"(FALSE ("P4")) -> ()
      }
      frame "ReadRN" {
        # "Read data read number of the PMT-Module"
        n88 = local read "RND"() -> (w320:i32)
        n89 = call "Read RN.vi"("RN"=w320, "handle"=w319) -> ("RN out"=w317:i32)  [unwired: 7 in, 2 out]
        n90 = local write "RND"(w317) -> ()
        n91 = local write "P6"(FALSE ("P4")) -> ()
      }
      frame "ReadSN" {
        # "Read data sweep number of the Motorized stage"
        n92 = Increment(x=w335) -> (x+1=w336:i32)
        n93 = local write "SN"(w336) -> ()
      }
      frame "CountStart" {
        # "Conter Start!"
        n94 = local read "Correction"() -> (w366:bool)
        n95 = Boolean To (0,1)(Boolean=w366) -> (0, 1=w368:i16)
        n96 = To Long Integer(number=w368) -> (32bit integer=w367:i32)
        n97 = call "Count Start.vi"("Correction"=w367, "handle"=w369) -> ()  [unwired: 8 in, 2 out]
      }
      frame "CountStop" {
        w385 = FALSE ("Start")
        # "Add Auto Sweep button local variable here"
        # "Conter Stop!"
        n98 = local write "Auto-Sweep"(w385) -> ()
        n99 = local write "Stop"(w385) -> ()
        n100 = local write "Start"(w385) -> ()
        n101 = call "Count Stop.vi"("handle"=w396) -> ()  [unwired: 9 in, 2 out]
        n102 = Build Array (concatenate)(w394, "ActiveSwitch") -> (w393:string[])
      }
      frame "ReadData" {
        # "Read Data...."
        n103 = stacked-sequence {
          seq-local: [_ w442 _] -> [_ _ w452]
          seq-local: [_ w441 _] -> [_ _ w453]
          tunnel: w421 -> [_ w447 _]
          tunnel: w420 -> [_ _ w455]
          tunnel: [_ _ w454] -> w419
          tunnel: [_ w437 _] -> w418
          tunnel: w417 -> [_ w440 _]
          frame #0 {
            # "DB Clear!"
            n104 = Initialize Array(u32 0, 16 ("次元サイズ")) -> (w434:u32[])
            n105 = local write "DB"(w434) -> ()
          }
          frame #1 {
            n106 = local read "OLD"() -> (w444:i32)
            n107 = local read "GN"() -> (w446:i32)
            n108 = local read "DB"() -> (w445:u32[])
            n109 = call "Read Data.vi"("OLD"=w444, "DataBuf"=w445, "GateNum"=w446, "handle"=w447) -> ("OLD out"=w443:i32, "DataBuf out"=w441:u32[], "GateNum out"=w439:i32, "function return"=w442:u32)  [unwired: 3 in, 1 out]
            n110 = local write "OLD"(w443) -> ()
            n111 = local write "GN"(w439) -> ()
            n112 = local write "DB"(w441) -> ()
            n113 = Build Array(w439) -> (w438:i32[])
            n114 = Build Array (concatenate)(w440, w438) -> (w437:i32[])
          }
          frame #2 {
            # "Check Over Rang !"
            # "ADD Data DIM"
            # "Pickup Tans Data!"
            n115 = To Long Integer(number=w452) -> (32bit integer=w450:i32)
            n116 = local read "OLD"() -> (w449:i32)
            n117 = Array Subset(array=w453, length=w450) -> (w451:u32[])  [unwired: 1 in]
            n118 = Not Equal To 0?(x=w449) -> (x != 0?=w448:bool)
            n119 = local write "OVL"(w448) -> ()
            n120 = Build Array (concatenate)(w455, w451) -> (w454:u32[])
            n121 = local write "Graph"(w454) -> ()
          }
        }
      }
      frame "AutoReadData" {
        # "Read Data...."
        n122 = stacked-sequence {
          tunnel: w461 -> [w486]
          tunnel: [w485] -> w460
          tunnel: w459 -> [w484]
          tunnel: w458 -> [w483]
          tunnel: w457 -> [w482]
          tunnel: [w481] -> w456
          frame #0 {
            n123 = Build Array (concatenate)(w483, w482) -> (w481:dbl[])
            n124 = Build Array (concatenate)(w484, w486) -> (w485:dbl[])
            n125 = local write "Sweep Graph"(w485) -> ()
          }
        }
      }
      frame "CountInit" {
        w497 = 0
        # "Auto"
        # "Clear Data DIM !"
        n126 = Initialize Array(w497, w497) -> (w495:i32[])
        n127 = Build Array("LockSwitch", "ReadRN", "CountStart", "ReadData", "CheckNumber") -> (w498:string[])
        n128 = Build Array (concatenate)(w504, w498) -> (w503:string[])
      }
      frame "AutoCount|nit!" {
        w532 = 0
        # "Clear Data DIM !"
        n129 = local read "SND"() -> (w519:i32)
        n130 = local read "SN"() -> (w524:i32)
        n131 = Increment(x=w519) -> (x+1=w520:i32)
        n132 = Initialize Array(w532, w532) -> (w531:i32[])
        n133 = Less?(x=w524, y=w520) -> (x < y?=w523:bool)
        n134 = case shown="True" w523 {
          tunnel: w522 -> [w548 w551]
          tunnel: [w546 w550] -> w521
          frame False {
            n135 = Build Array("AutoReadData", "AutoCheckNumber") -> (w547:string[])
            n136 = Build Array (concatenate)(w548, w547) -> (w546:string[])
          }
          frame True {
            n137 = Build Array("LockSwitch", "ReadRN", "CountStart", "ReadData", "AutoCheckNumber") -> (w557:string[])
            n138 = Build Array (concatenate)(w551, w557) -> (w550:string[])
          }
        }
      }
      frame "CheckNumber" {
        # "Add append"
        # "Add Case Strucutre outside\nsimilar to GN,"
        # "Check RN and Data lenbgth,Stop Switch ......"
        n139 = local read "Stop"() -> (w568:bool)
        n140 = local read "GN"() -> (w569:i32)
        n141 = Decrement(x=w571) -> (x-1=w570:i32)
        n142 = Less?(x=w569, y=w570) -> (x < y?=w575:bool)
        n143 = case shown="False" w575 {
          tunnel: [w590 w592] -> w572
          tunnel: w568 -> [_ w591]
          frame False {
            # "\"MotorJog\"; here"
            # "Move \"Active Swith\" to False Condition of Position Number"
            # "Add \"AutoExport Run\" here"
            n144 = local write "Start"(FALSE ("Start")) -> ()
            n145 = Build Array("CountStop", "ActiveSwitch") -> (w590:string[])
          }
          frame True {
            n146 = case shown="False" w591 {
              tunnel: [w594 w596] -> w592
              frame False {
                n147 = Build Array("ReadData", "CheckNumber") -> (w594:string[])
              }
              frame True {
                n148 = Build Array("CountStop") -> (w596:string[])
              }
            }
          }
        }
        n149 = Build Array (concatenate)(w573, w572) -> (w574:string[])
      }
      frame "AutoCheckNumber" {
        # "Add append"
        # "Add Case Strucutre outside\nsimilar to GN,"
        # "Check RN and Data lenbgth,Stop Switch ......"
        n150 = local read "Stop"() -> (w611:bool)
        n151 = local read "SND"() -> (w600:i32)
        n152 = local read "SN"() -> (w604:i32)
        n153 = Less?(x=w604, y=w600) -> (x < y?=w603:bool)
        n154 = case shown="False" w603 {
          tunnel: [w628 w638] -> w613
          tunnel: w612 -> [_ w637]
          tunnel: w611 -> [_ w634]
          tunnel: [TRUE w633] -> w606
          frame False {
            w632 = FALSE ("Start")
            n155 = local write "Auto-Sweep"(w632) -> ()
            n156 = local write "Start"(w632) -> ()
            n157 = Build Array("CountStop", "AutoExportSweep", "ActiveSwitch") -> (w628:string[])
          }
          frame True {
            n158 = local read "GN"() -> (w635:i32)
            n159 = Decrement(x=w637) -> (x-1=w636:i32)
            n160 = Less?(x=w635, y=w636) -> (x < y?=w639:bool)
            n161 = case shown="False" w639 {
              tunnel: [w641 w657] -> w638
              tunnel: w634 -> [w642 w656]
              tunnel: [w640 w655] -> w633
              frame False {
                # "\"MotorJog\"; here"
                # "Move \"Active Swith\" to False Condition of Position Number"
                # "Add \"AutoExport Run\" here"
                n162 = case shown="False" w642 {
                  tunnel: [w648 w653] -> w641
                  tunnel: [FALSE TRUE] -> w640
                  frame False {
                    n163 = Build Array("CountStop", "AutoExportRun", "AutoReadData", "ReadSN", "MotorJog", "AutoCount|nit!") -> (w648:string[])
                  }
                  frame True {
                    n164 = local write "Auto-Sweep"(TRUE) -> ()
                    n165 = Build Array("CountStop") -> (w653:string[])
                  }
                }
              }
              frame True {
                n166 = case shown="False" w656 {
                  tunnel: [w660 w664] -> w657
                  tunnel: [FALSE TRUE] -> w655
                  frame False {
                    n167 = Build Array("ReadData", "AutoCheckNumber") -> (w660:string[])
                  }
                  frame True {
                    n168 = Build Array("CountStop") -> (w664:string[])
                    n169 = local write "Auto-Sweep"(TRUE) -> ()
                  }
                }
              }
            }
          }
        }
        n170 = Build Array (concatenate)(w614, w613) -> (w615:string[])
      }
      frame "Export" {
        # "For Auto Export also add mean waveform"
        # "Get mean Data into 1D array Shift register for waveform"
        # "Gate Number is just number of count measurements"
        # "time...using array size"
        # "time...using array size"
        n171 = Array Size(array=w682) -> (size(s)=w694:i32)
        n172 = for {
          N: w694 -> [_]
          tunnel: [w709] -> w681 mode=indexing
          i -> [w711]
          n173 = local read "ITD"() -> (w713:i32)
          n174 = Add(x=1, y=w711) -> (x+y=w712:i32)
          n175 = Multiply(x=w713, y=w712) -> (x*y=w709:i32)
        }
        n176 = call <vilib>:"Std Deviation and Variance.vi"("X"=w682) -> ("mean"=w675:dbl, "standard deviation"=w674:dbl)  [unwired: 1 in, 1 out]
        n177 = Build Array(w675, w674) -> (w673:dbl[])
        n178 = Build Array(w677, w681, w682) -> (w692:u32[][])
        n179 = call-poly <vilib>:"Write Delimited Spreadsheet.vi"("1D data"=string[] ["Gate  No.", "Time [ms]", "Counts"], "append to file? (new file:F)"=FALSE, "transpose? (no:F)"=FALSE) -> ("new file path (Not A Path if cancelled)"=w691:path)  [unwired: 11 in, 1 out]
        n180 = call-poly <vilib>:"Write Delimited Spreadsheet.vi"("file path (dialog if empty)"=w691, "2D data"=w692, "append to file? (new file:F)"=TRUE, "transpose? (no:F)"=TRUE) -> ("new file path (Not A Path if cancelled)"=w687:path)  [unwired: 10 in, 1 out]
        n181 = call-poly <vilib>:"Write Delimited Spreadsheet.vi"("file path (dialog if empty)"=w687, "1D data"=string[] ["Mean", "Std. Dev."], "append to file? (new file:F)"=TRUE, "transpose? (no:F)"=FALSE) -> ("new file path (Not A Path if cancelled)"=w683:path)  [unwired: 10 in, 1 out]
        n182 = call-poly <vilib>:"Write Delimited Spreadsheet.vi"("file path (dialog if empty)"=w683, "1D data"=w673, "append to file? (new file:F)"=TRUE, "transpose? (no:F)"=FALSE) -> ()  [unwired: 10 in, 2 out]
        n183 = local write "Export"(FALSE) -> ()
      }
      frame "AutoExportRun" {
        # "For Auto Export also add mean waveform"
        # "Get mean Data into 1D array Shift register for waveform"
        # "Gate Number is just number of count measurements"
        # "time...using array size"
        n184 = Array Size(array=w731) -> (size(s)=w733:i32)
        n185 = for {
          N: w733 -> [_]
          tunnel: [w775] -> w730 mode=indexing
          i -> [w777]
          n186 = local read "ITD"() -> (w779:i32)
          n187 = Add(x=1, y=w777) -> (x+y=w778:i32)
          n188 = Multiply(x=w779, y=w778) -> (x*y=w775:i32)
        }
        n189 = flat-sequence {
          tunnel: w722 -> [w774]
          tunnel: [w770] -> w721
          frame #0 {
            n190 = local read "SS"() -> (w773:i32)
            n191 = Multiply(x=w774, y=w773) -> (x*y=w771:i32)
            n192 = local read "SP"() -> (w772:i32)
            n193 = Add(x=w772, y=w771) -> (x+y=w770:i32)
          }
        }
        n194 = call <vilib>:"Std Deviation and Variance.vi"("X"=w731) -> ("mean"=w725:dbl, "standard deviation"=w715:dbl)  [unwired: 1 in, 1 out]
        n195 = Build Array(w725, w715) -> (w728:dbl[])
        n196 = Number To Decimal String(number=w721) -> (decimal integer string=w720:string)  [unwired: 1 in]
        n197 = Build Array(w717, w730, w731) -> (w732:u32[][])
        n198 = Build Array (concatenate)(string[] ["Angle (deg)"], w720) -> (w718:string[])
        n199 = case shown="True" "Save All Gate Data" {
          tunnel: w732 -> [_ w768]
          tunnel: w728 -> [_ w755]
          tunnel: [w748 w754] -> w727
          tunnel: w723 -> [w748 w753]
          tunnel: w718 -> [_ w749]
          frame False {
          }
          frame True {
            # "time...using array size"
            n200 = call-poly <vilib>:"Write Delimited Spreadsheet.vi"("file path (dialog if empty)"=w753, "1D data"=w749, "append to file? (new file:F)"=TRUE, "transpose? (no:F)"=FALSE) -> ("new file path (Not A Path if cancelled)"=w752:path)  [unwired: 10 in, 1 out]
            n201 = call-poly <vilib>:"Write Delimited Spreadsheet.vi"("file path (dialog if empty)"=w752, "1D data"=string[] ["Gate  No.", "Time [ms]", "Counts"], "append to file? (new file:F)"=TRUE, "transpose? (no:F)"=FALSE) -> ("new file path (Not A Path if cancelled)"=w767:path)  [unwired: 10 in, 1 out]
            n202 = call-poly <vilib>:"Write Delimited Spreadsheet.vi"("file path (dialog if empty)"=w767, "2D data"=w768, "append to file? (new file:F)"=TRUE, "transpose? (no:F)"=TRUE) -> ("new file path (Not A Path if cancelled)"=w763:path)  [unwired: 10 in, 1 out]
            n203 = call-poly <vilib>:"Write Delimited Spreadsheet.vi"("file path (dialog if empty)"=w763, "1D data"=string[] ["Mean", "Std. Dev."], "append to file? (new file:F)"=TRUE, "transpose? (no:F)"=FALSE) -> ("new file path (Not A Path if cancelled)"=w759:path)  [unwired: 10 in, 1 out]
            n204 = call-poly <vilib>:"Write Delimited Spreadsheet.vi"("file path (dialog if empty)"=w759, "1D data"=w755, "append to file? (new file:F)"=TRUE, "transpose? (no:F)"=FALSE) -> ("new file path (Not A Path if cancelled)"=w754:path)  [unwired: 10 in, 1 out]
          }
        }
        n205 = local write "Export"(FALSE) -> ()
      }
      frame "AutoExportSweep" {
        w789 = 0
        w788 = 0.0
        # "Gate Number is just number \nof count measurements"
        # "For Auto Export also add mean waveform"
        # "Get mean Data into 1D array Shift register for waveform"
        # "time...using array size"
        # "time...using array size"
        n206 = Array Size(array=w792) -> (size(s)=w808:i32)
        n207 = for {
          N: w808 -> [_]
          tunnel: [w836] -> w800 mode=indexing
          i -> [w833]
          n208 = local read "SS"() -> (w837:i32)
          n209 = Multiply(x=w837, y=w833) -> (x*y=w834:i32)
          n210 = local read "SP"() -> (w835:i32)
          n211 = Add(x=w835, y=w834) -> (x+y=w836:i32)
        }
        n212 = call <vilib>:"Std Deviation and Variance.vi"("X"=w792) -> ("mean"=w793:dbl, "standard deviation"=w785:dbl)  [unwired: 1 in, 1 out]
        n213 = Initialize Array(w788, w789) -> (w790:dbl[])
        n214 = Initialize Array(w788, w789) -> (w787:dbl[])
        n215 = Build Array(w793, w785) -> (w781:dbl[])
        n216 = Build Array(w800, w792, w786) -> (w806:dbl[][])
        n217 = call-poly <vilib>:"Write Delimited Spreadsheet.vi"("file path (dialog if empty)"=w794, "1D data"=string[] ["Angle", "CountsMean", "CountsSTD"], "append to file? (new file:F)"=TRUE, "transpose? (no:F)"=FALSE) -> ("new file path (Not A Path if cancelled)"=w805:path)  [unwired: 10 in, 1 out]
        n218 = call-poly <vilib>:"Write Delimited Spreadsheet.vi"("file path (dialog if empty)"=w805, "2D data"=w806, "append to file? (new file:F)"=TRUE, "transpose? (no:F)"=TRUE) -> ("new file path (Not A Path if cancelled)"=w802:path)  [unwired: 10 in, 1 out]
        n219 = case shown="False" FALSE {
          tunnel: w802 -> [w823 w831]
          tunnel: w781 -> [_ w828]
          tunnel: [w823 w825] -> w780
          frame False {
          }
          frame True {
            n220 = call-poly <vilib>:"Write Delimited Spreadsheet.vi"("file path (dialog if empty)"=w831, "1D data"=string[] ["Mean", "Std. Dev."], "append to file? (new file:F)"=TRUE, "transpose? (no:F)"=FALSE) -> ("new file path (Not A Path if cancelled)"=w829:path)  [unwired: 10 in, 1 out]
            n221 = call-poly <vilib>:"Write Delimited Spreadsheet.vi"("file path (dialog if empty)"=w829, "1D data"=w828, "append to file? (new file:F)"=TRUE, "transpose? (no:F)"=FALSE) -> ("new file path (Not A Path if cancelled)"=w825:path)  [unwired: 10 in, 1 out]
          }
        }
        n222 = local write "Export"(FALSE) -> ()
      }
      frame "AutoSweep" {
        w842 = 0
        # "1. Create a file path (Send two strings, \"SetPosition\" and \"AutoCount|nit!\")\n2. Send to \"SetPosition\"\n2.1. Will create a Position Number Shift register\n2.2. Move stage to initial position, allow time to complete movement or add delay\n3. Send to \"AutoCount|nit!\"\n3.1. \"AutoCount|nit!\" is clone of \"Count|nit!\" but sends to \"AutoCheckNumber\", not \"CheckNumber\n3.1.1. \"AutoCheckNumber\" will check if end position, or run condition is met then send \"CountStop\" and \"ActiveSwitch\"\n3.1.2. \"AutoCheck Number\" will allow \"CountStop\" to be sent via Stop Boolean\n3.1.3. \"AutoCheckNumber\" will upon END of one run will run \"AutoExportRun\" to set file path\n3.1.3.1. \"AutoExportRun\" will add a data point to Mean Waveform after Count Stop\n3.1.4. \"AutoCheckNumber\" will upon END of sweep will run \"AutoExportSweep\" then issue \"ActiveSwitch\"\n3.1.4.1. \"AutoExportSweep\" will append final Mean Sweep waveform to file path before \"CountStop\";\"ActiveSwitch\"\n4. If End condition not met; \"MotorJog\"; \"AutoCount|nit!\"....repeats\n4.1. Will move to next position by set increment, with .net code, add delay to allow it to arrive at position"
        # "Create a File path here\nSend switch case string \"SetPosition\", which has a position number switch register"
        # "1.Position Set, create a file path\n2. Count|nit!---duplicate and create auto counter, add read sweep data for auto read\n2.0.1Checknumber end, change active switch to Auto export\n3. Auto Export ... need to make \n3.0.2Auto Export end, send to read sweep data (mean, stdev for per sweep)\n3.Export\n4.check end position, check end condition met\n5.met>end;not end >continue\n6. Jog motor\n7.repeat from 2."
        # "Create Motor Controls for setting Homing, Step size for angle, idle time(if required),"
        n223 = local write "SN"(w842) -> ()
        n224 = call-poly <vilib>:"Write Delimited Spreadsheet.vi"("append to file? (new file:F)"=FALSE) -> ("new file path (Not A Path if cancelled)"=w841:path)  [unwired: 13 in, 1 out]
        n225 = Build Array("SetPosition", "AutoCount|nit!") -> (w847:string[])
        n226 = Build Array (concatenate)(w845, w847) -> (w844:string[])
      }
      frame "MotorJog" {
        # "Move position by set increment"
        # "Add a test Jog?"
        # "Put thor labs net code here"
        n227 = stacked-sequence {
          tunnel: w873 -> [w895 w900]
          frame #0 {
            n228 = local read "SSD"() -> (w894:i32)
            n229 = invoke class="KCubeDCServo" method="MoveRelative"(reference=w895, "direction"=1, "stepSize"=w894, "waitTimeout"=0) -> ()  [unwired: 2 in, 6 out]
            n230 = local read "WT"() -> (w892:i32)
            n231 = Wait (ms)(milliseconds to wait=w892) -> ()  [unwired: 1 out]
          }
          frame #1 {
            n232 = invoke class="KCubeDCServo" method="GetPositionCounter"(reference=w900) -> ("GetPositionCounter"=w898:i32)  [unwired: 2 in, 2 out]
            n233 = Divide(x=w898, y=1919.6418578623338) -> (x/y=w896:dbl)
            n234 = Wait (ms)(milliseconds to wait=50) -> ()  [unwired: 1 out]
            n235 = local write "PC"(w896) -> ()
          }
        }
        n236 = local write "P8"(FALSE) -> ()
      }
      frame "SetPosition" {
        n237 = stacked-sequence {
          tunnel: w907 -> [w926 w929 w934]
          frame #0 {
            n238 = local read "SPD"() -> (w925:i32)
            n239 = invoke class="KCubeDCServo" method="SetMoveAbsolutePosition"(reference=w926, "position"=w925) -> ()  [unwired: 2 in, 4 out]
          }
          frame #1 {
            n240 = invoke class="KCubeDCServo" method="MoveAbsolute"(reference=w929, "waitTimeout"=0) -> ()  [unwired: 2 in, 4 out]
            n241 = local read "WT"() -> (w928:i32)
            n242 = Wait (ms)(milliseconds to wait=w928) -> ()  [unwired: 1 out]
          }
          frame #2 {
            n243 = invoke class="KCubeDCServo" method="GetPositionCounter"(reference=w934) -> ("GetPositionCounter"=w931:i32)  [unwired: 2 in, 2 out]
            n244 = Divide(x=w931, y=1919.6418578623338) -> (x/y=w930:dbl)
            n245 = local write "PC"(w930) -> ()
            n246 = Wait (ms)(milliseconds to wait=50) -> ()  [unwired: 1 out]
          }
        }
      }
      frame "", "Idle" {
        n247 = event shown="[12] \"Auto-Sweep\": Value Change" {
          selector: _ -> [_ _ _ _ _ _ _ _ _ _ _ _ _]
          dyn-events: _ -> [_ _ _ _ _ _ _ _ _ _ _ _ _]
          timeout: _ -> [_ _ _ _ _ _ _ _ _ _ _ _ _]
          tunnel: w948 -> [w963 w966 w969 w973 w977 w981 w985 w989 w992 w994 w997 w1000 w1003]
          tunnel: [w961 w965 w968 w972 w976 w980 w984 w988 w991 w993 w996 w999 w1004] -> w946
          event Menu Selection (User) {
            n248 = event-data() -> ("ItemTag"=w962:string)  [unwired: 1 out]
            n249 = Build Array (concatenate)(w963, w962) -> (w961:string[])
          }
          event "EXIT": Value Change {
            n250 = event-data() -> ()  [unwired: 7 out]
            n251 = Build Array (concatenate)(w966, "Exit") -> (w965:string[])
          }
          event "P1": Value Change {
            n252 = event-data() -> ()  [unwired: 7 out]
            n253 = Build Array (concatenate)(w969, "SetPower") -> (w968:string[])
          }
          event "P2": Value Change {
            n254 = event-data() -> ()  [unwired: 7 out]
            n255 = Build Array (concatenate)(w973, "ReadPower") -> (w972:string[])
            n256 = Wait (ms)(milliseconds to wait=u32 200 ("ミリ秒待機時間")) -> ()  [unwired: 1 out]
          }
          event "P3": Value Change {
            n257 = event-data() -> ()  [unwired: 7 out]
            n258 = Build Array (concatenate)(w977, "SetIT") -> (w976:string[])
            n259 = Wait (ms)(milliseconds to wait=u32 200 ("ミリ秒待機時間")) -> ()  [unwired: 1 out]
          }
          event "P4": Value Change {
            n260 = event-data() -> ()  [unwired: 7 out]
            n261 = Build Array (concatenate)(w981, "ReadIT") -> (w980:string[])
            n262 = Wait (ms)(milliseconds to wait=u32 200 ("ミリ秒待機時間")) -> ()  [unwired: 1 out]
          }
          event "P5": Value Change {
            n263 = event-data() -> ()  [unwired: 7 out]
            n264 = Build Array (concatenate)(w985, "SetRN") -> (w984:string[])
            n265 = Wait (ms)(milliseconds to wait=u32 200 ("ミリ秒待機時間")) -> ()  [unwired: 1 out]
          }
          event "P6": Value Change {
            n266 = event-data() -> ()  [unwired: 7 out]
            n267 = Build Array (concatenate)(w989, "ReadRN") -> (w988:string[])
            n268 = Wait (ms)(milliseconds to wait=u32 200 ("ミリ秒待機時間")) -> ()  [unwired: 1 out]
          }
          event "Start": Value Change {
            n269 = event-data() -> ()  [unwired: 7 out]
            n270 = Build Array (concatenate)(w992, "CountInit") -> (w991:string[])
          }
          event "Export": Value Change {
            n271 = event-data() -> ()  [unwired: 7 out]
            n272 = Build Array (concatenate)(w994, "Export") -> (w993:string[])
          }
          event "P7": Value Change {
            n273 = event-data() -> ()  [unwired: 7 out]
            n274 = Build Array (concatenate)(w997, "SetStepProp") -> (w996:string[])
          }
          event "P8": Value Change {
            n275 = event-data() -> ()  [unwired: 7 out]
            n276 = Build Array (concatenate)(w1000, "MotorJog") -> (w999:string[])
          }
          event "Auto-Sweep": Value Change {
            n277 = event-data() -> ()  [unwired: 7 out]
            n278 = Build Array (concatenate)(w1003, "AutoSweep") -> (w1004:string[])
            n279 = Wait (ms)(milliseconds to wait=200) -> ()  [unwired: 1 out]
          }
        }
        n280 = Build Array (concatenate)("", w946) -> (w945:string[])
      }
      frame "Error", Default {
        n281 = Concatenate Strings("Error  Case Name .....", "\r\n", w1015) -> (w1017:string)
        n282 = One Button Dialog(message=w1017) -> (true=w1016:bool)  [unwired: 1 out]
        n283 = stacked-sequence {
          tunnel: w1016 -> [_]
          frame #0 {
            n284 = Stop() -> ()  [unwired: 1 out]
          }
        }
      }
      frame "Exit" {
        # "See you again ......"
        n285 = call "Close.vi"("Handle"=w1043) -> ()  [unwired: 9 in, 2 out]
      }
    }
    n286 = Divide(x=w18, y=1919.6418578623338) -> (x/y=w17:dbl)
    n287 = local write "PC"(w17) -> ()
    n288 = call "SM_CaseErase.vi"("Input"=w43) -> ("Output"=w42:string[])  [unwired: 10 out]
  }
  n289 = invoke class="KCubeDCServoControl" method="CloseDevice"(reference=w6) -> ()  [unwired: 2 in, 3 out]
